vi "3D FIELD SWEEP with feedback, logging, both modes, starting step, and 1D sweep.vi"() -> ()   [LabVIEW 2018]
doc: "This example performs a serial port write and a serial port read. The parameters set for the serial port must match the parameters of the connected instrument or device. The VISA Configure Serial Port VI sets the configuration parameters. The front panel displays the controls used to configure the basic parameters, such as baud rate, data bits, and parity. The VI passes the VISA resource name to other VIs that perform operations on that VISA resource. The VISA Write function sends a command to the serial device and the VISA Read function returns data based on the command. The VISA Close function then closes the reference to the serial device. It is important to close the reference; otherwise, further communication through that port might not be possible."
uses:
  Program Files/National Instruments/LabVIEW 2018/examples/Instrument IO/Serial/support/Serial - Settings.ctl
  <vilib>/Instr/_visa.llb/VISA Configure Serial Port (Instr).vi
  <vilib>/Utility/file.llb/Write Delimited Spreadsheet (string).vi
panel:
  out "Magnetic field z [µT]":dbl
  out "Magnetic field y [µT]":dbl
  out "Magnetic field x [µT]":dbl
  out "Magnetic field strength [µT]":dbl
  in  "Direction field sweep":string(combo)
  in  "Minimum value B [µT]":dbl
  in  "Maximum value B [µT]":dbl
  in  "START":bool
  in  "Number of steps":dbl
  out "Current has stabilized":bool
  in  "Next iteration 2":bool
  in  "Starting step":dbl
  out "Current has stabilized":bool
  out "Current has stabilized":bool
  in  "Next iteration":bool
  in  "file path (use dialog)":path
  in  "Start":bool
  out "Start time 2":timestamp
  out "Angle \"phi\"":dbl
  out "Current iteration":i32
  in  "Number of steps":dbl
  in  "Angle theta [degrees]":dbl
  in  "Magnetic field strength [µT]":dbl
  in  "Octant":string(combo)
  in  "Sweep plane & fixed axis":string(combo)
  in  "OFF":bool
  in  "OK Button":bool
  in  "Magnetic field strength z [µT]":dbl
  in  "Magnetic field strength y [µT]":dbl
  in  "Magnetic field strength x [µT]":dbl
  in  "Static or field sweep?":string(combo)
  in  "Serial Settings":T1={"baud rate"=9600, "data bits"=8, "parity"=enum."None", "stop bits"=10, "flow control"=0} {"flow control" items=["None"=0, "XON/XOFF"=1, "RTS/CTS"=2, "DTR/DSR"=4]; "stop bits" items=["1.0"=10, "1.5"=15, "2.0"=20]; "data bits" min=5 max=8 step=1; "baud rate" items=["75"=75, "110"=110, "134"=134, "150"=150, "300"=300, "600"=600, "1200"=1200, "1800"=1800, "2400"=2400, "4800"=4800, "7200"=7200, "9600"=9600, "14400"=14400, "19200"=19200, "28800"=28800, "38400"=38400, "56000"=56000, "57600"=57600, "115200"=115200, "128000"=128000, "230400"=230400]}
  in  "VISA resource name":refnum<visa-resource-name>="COM1"
  # "Static field"
  # "1D magnitude sweep"
  # "Settings"
  # "3D field sweep"
  # "About the 3D field sweep"
  # "A onstant-magnitude, fixed-tilt, azimuthal sweep of a 3D vector is performed.\nThe mag,netic field vector is angled away from a fixed axis by a certain angle \"phi\". It then makes a circular motion around that fixed axis, eventually tracing out a full cone.\nYou choose a plane of variation ( x–y, x–z, or y–z) and hold one direction constant (e.g., z).  The sweep is performed clockwise, as seen from the origin."
  # "Must be a csv comma delimited excell file."
  # "How to connect the cables"
  # "Current state"
  # "Current state"
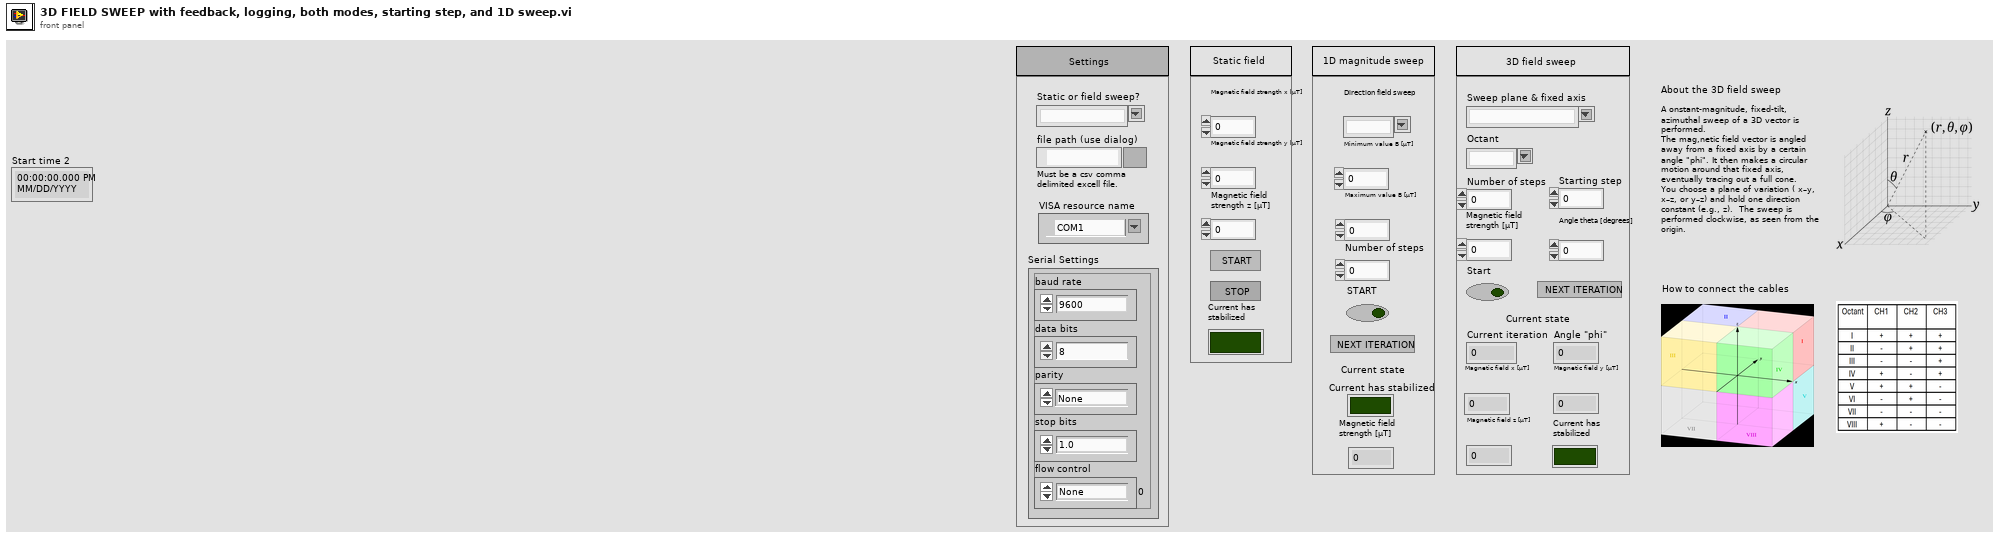
[diagram p1: front panel]
types:
  T1 = typedef "Serial - Settings.ctl" = cluster{"baud rate":u32, "data bits":u16, "parity":enum16{"None", "Odd", "Even", "Mark", "Space"}, "stop bits":u16, "flow control":u16}
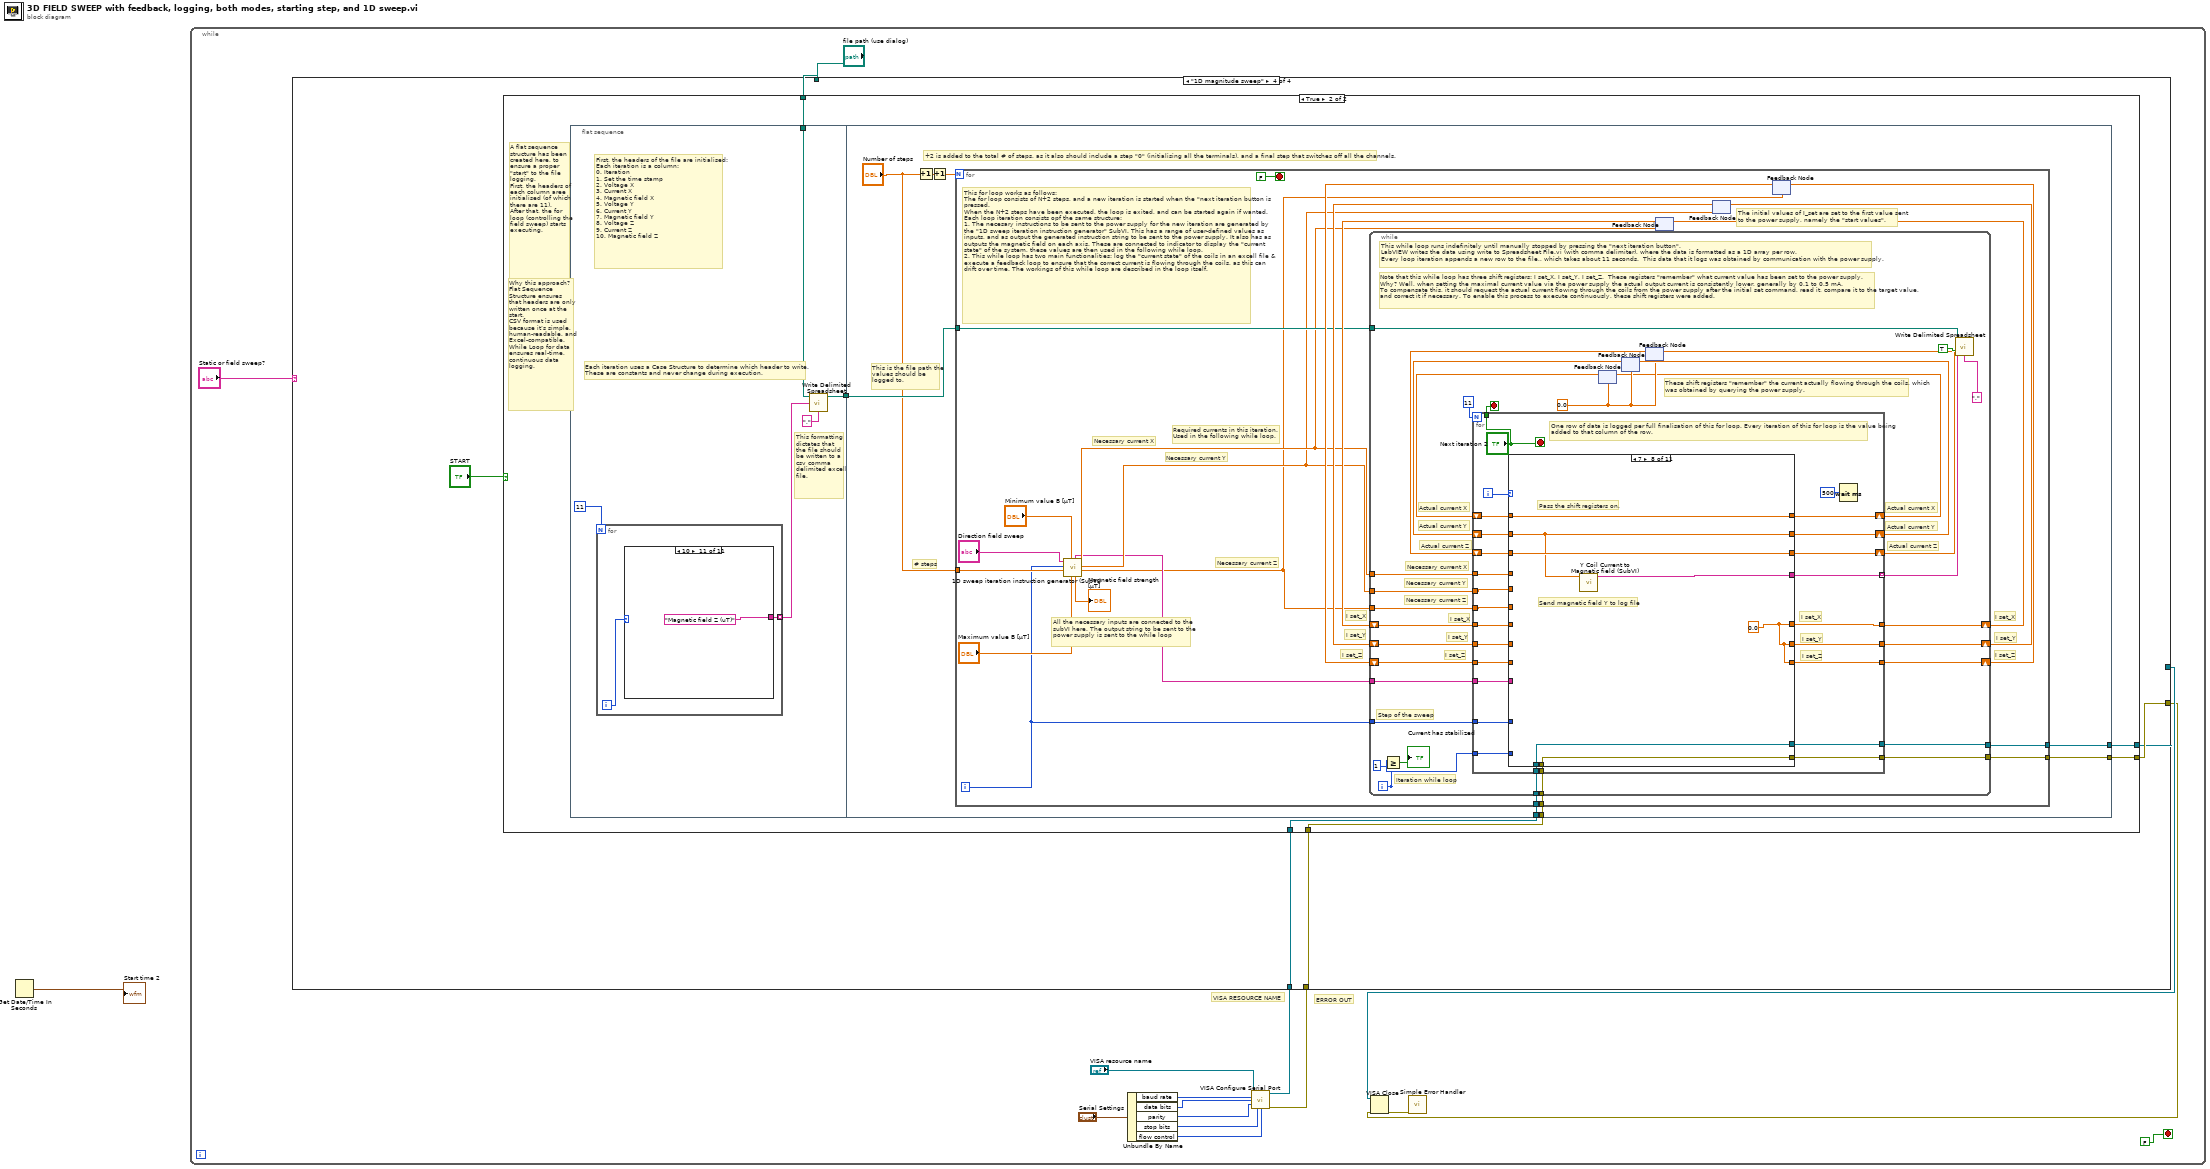
[diagram p0: block diagram]
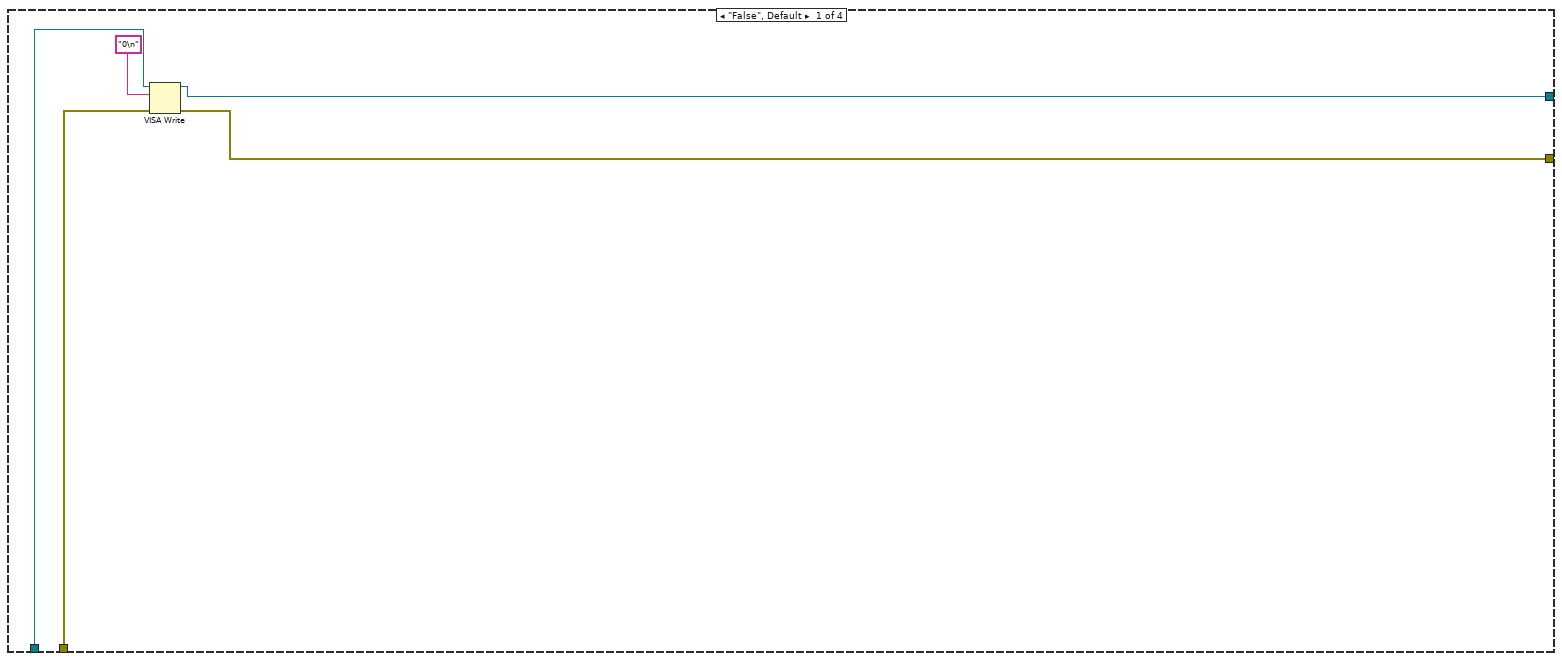
[diagram p2: hidden frame]
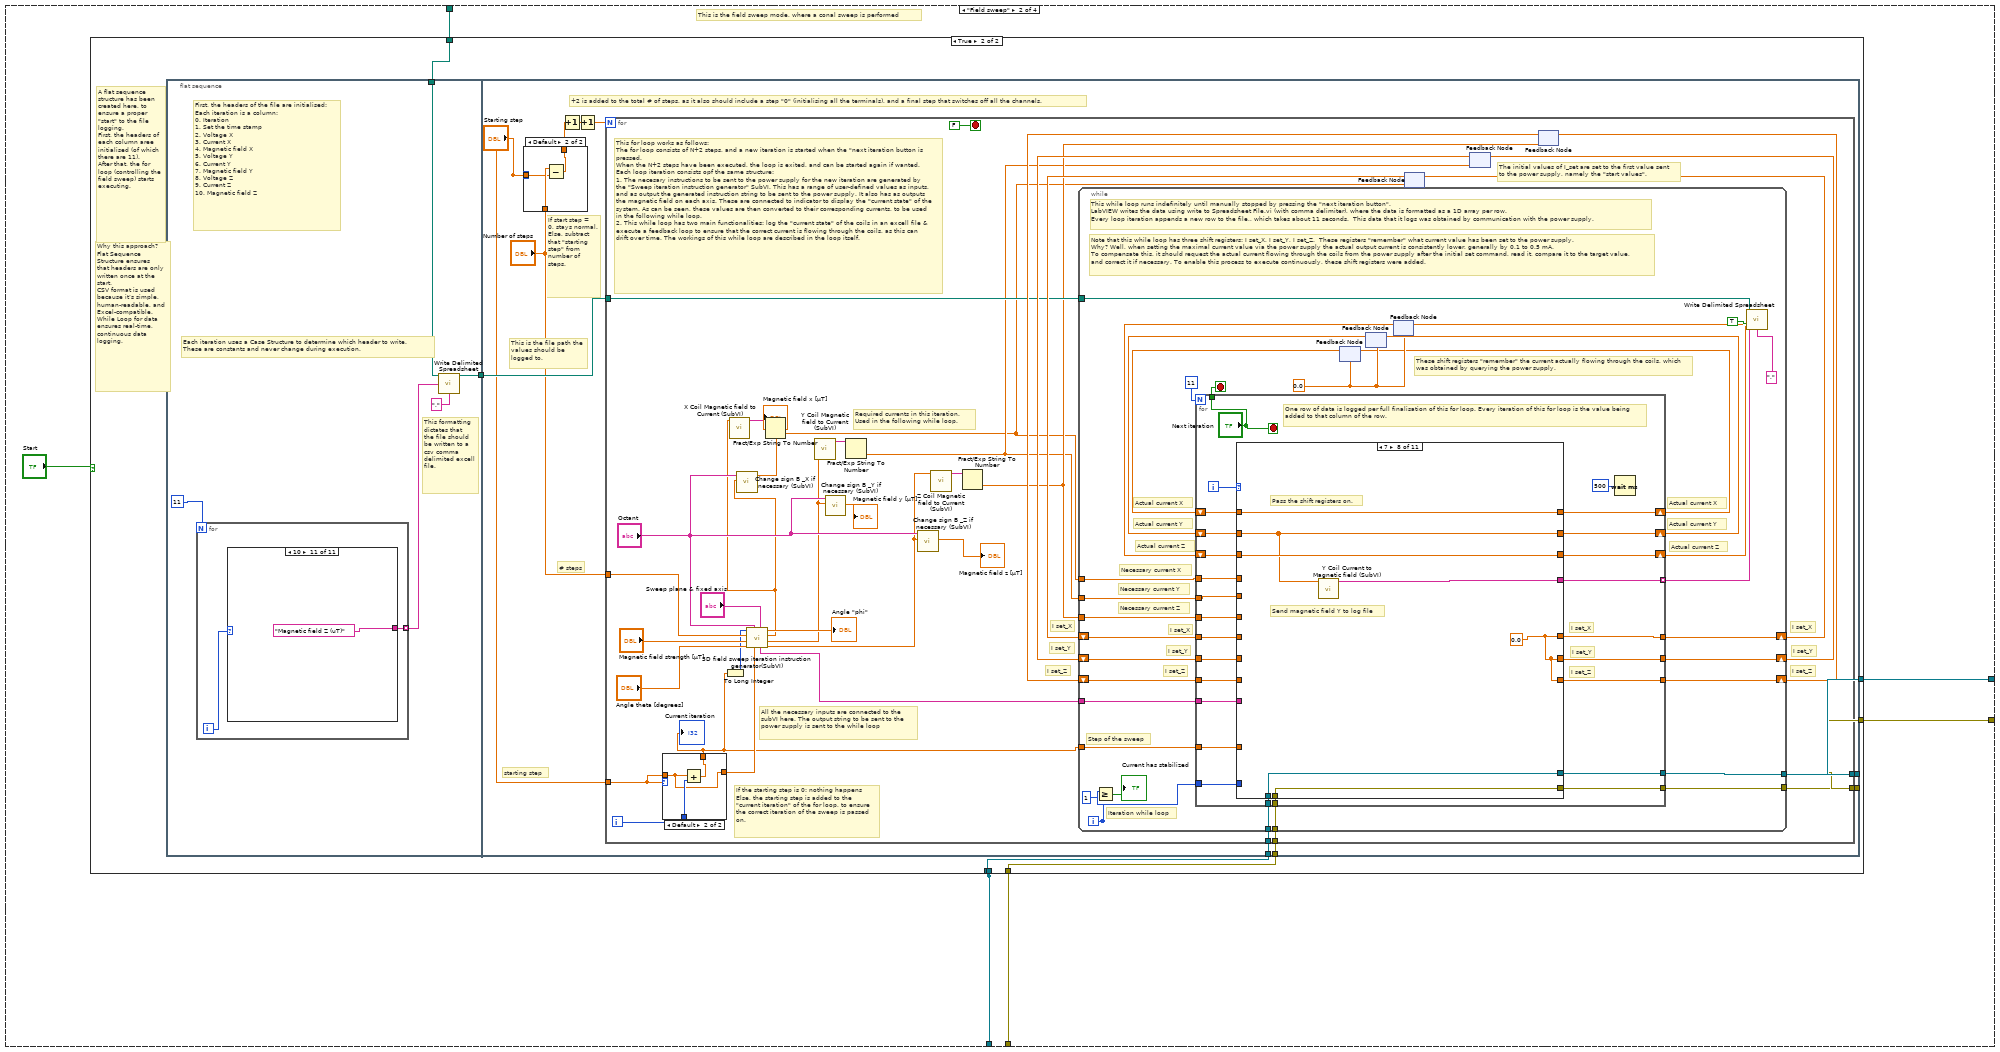
[diagram p3: hidden frame]
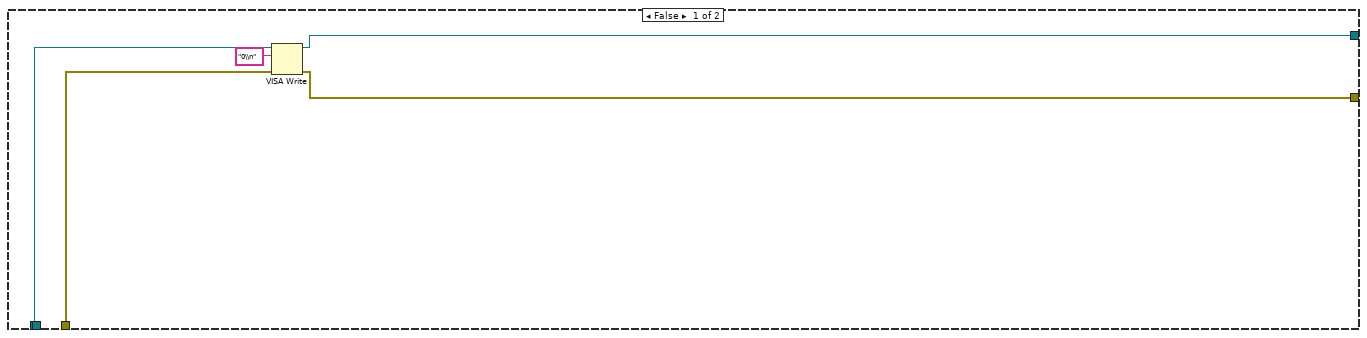
[diagram p4: hidden frame]
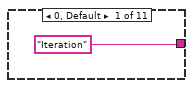
[diagram p5: hidden frame]
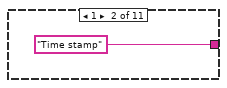
[diagram p6: hidden frame]
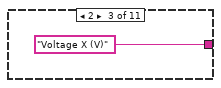
[diagram p7: hidden frame]
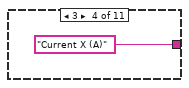
[diagram p8: hidden frame]
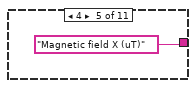
[diagram p9: hidden frame]
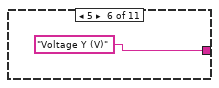
[diagram p10: hidden frame]
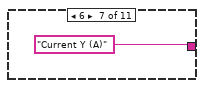
[diagram p11: hidden frame]
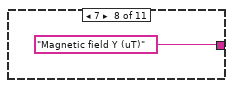
[diagram p12: hidden frame]
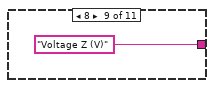
[diagram p13: hidden frame]
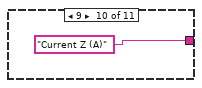
[diagram p14: hidden frame]
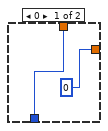
[diagram p16: hidden frame]
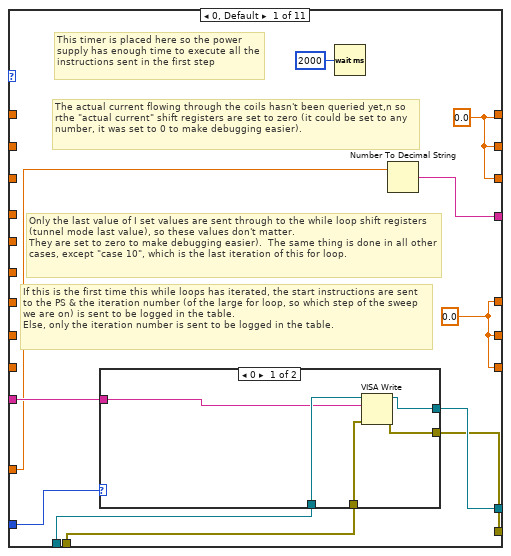
[diagram p17: hidden frame]
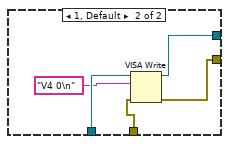
[diagram p18: hidden frame]
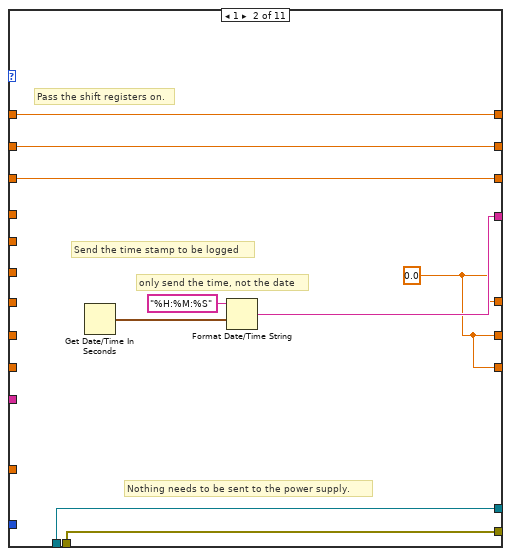
[diagram p19: hidden frame]
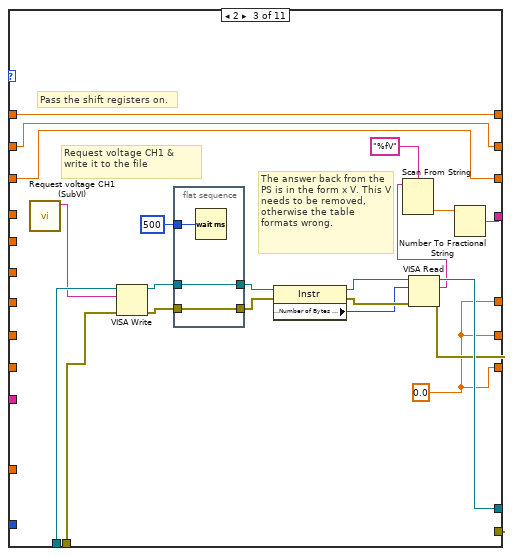
[diagram p20: hidden frame]
diagram:
  n1 = Get Date/Time In Seconds() -> (seconds since 1Jan1904=→"Start time 2":timestamp)
  n2 = while {
    stop <- FALSE stop-if-true
    # "VISA RESOURCE NAME"
    # "ERROR OUT"
    n3 = Unbundle By Name("Serial Settings") -> ("baud rate"=w13:u32, "data bits"=w2:u16, "parity"=w12:enum16{"None", "Odd", "Even", "Mark", "Space"}, "stop bits"=w11:u16, "flow control"=w10:u16)
    n4 = call-poly "VISA Configure Serial Port"("VISA resource name"="VISA resource name", "baud rate (9600)"=w13, "data bits (8)"=w2, "parity (0:none)"=w12, "stop bits (10: 1 bit)"=w11, "flow control (0:none)"=w10) -> ("VISA resource name out"=w3:refnum<visa-resource-name>, "error out"=w9:errorcluster)  [unwired: 3 in, 5 out]
    n5 = case shown="\"1D magnitude sweep\"" "Static or field sweep?" {
      tunnel: [w17 w26 w424 w793] -> w7
      tunnel: w3 -> [w19 w24 w421 w795]
      tunnel: w9 -> [w20 w25 w425 w794]
      tunnel: [w18 w27 w423 w792] -> w8
      tunnel: "file path (use dialog)" -> [_ w22 w420 w797]
      frame "False", Default {
        n6 = VISA Write(VISA resource name=w19, write buffer="0\n", error in (no error)=w20) -> (VISA resource name out=w18:refnum<visa-resource-name>, error out=w17:errorcluster)  [unwired: 1 out]
      }
      frame "Field sweep" {
        # "This is the field sweep mode, where a conal sweep is performed"
        n7 = case shown="True" "Start" {
          tunnel: [w32 w36] -> w27
          tunnel: [w31 w35] -> w26
          tunnel: w24 -> [w29 w38]
          tunnel: w25 -> [w30 w37]
          tunnel: w24 -> [_ _]
          tunnel: w22 -> [_ w33]
          frame False {
            n8 = VISA Write(VISA resource name=w29, write buffer="0\\n", error in (no error)=w30) -> (VISA resource name out=w32:refnum<visa-resource-name>, error out=w31:errorcluster)  [unwired: 1 out]
          }
          frame True {
            # "Why this approach?\nFlat Sequence Structure ensures that headers are only written once at the start.\nCSV format is used because it’s simple, human-readable, and Excel-compatible.\nWhile Loop for data ensures real-time, continuous data logging."
            # "A flat sequence structure has been created here, to ensure a proper \"start\" to the file logging. \nFirst, the headers of each column aree initialised (of which there are 11). \nAfter that, the for loop (controlling the field sweep) starts executing."
            n9 = flat-sequence {
              tunnel: w33 -> [w40]
              tunnel: [w39] -> w34
              tunnel: w38 -> [w64]
              tunnel: w37 -> [w63]
              tunnel: [w62] -> w36
              tunnel: [w61] -> w35
              tunnel: w34 -> [w60]
              frame #0 {
                # "Each iteration uses a Case Structure to determine which header to write.\nThese are constants and never change during execution."
                # "This formatting dictates that the file should be written to a csv comma delimited excell file."
                # "First, the headers of the file are initialised:\nEach iteration is a column:\n0. Iteration\n1. Set the time stamp\n2. Voltage X\n3. Current X\n4. Magnetic field X\n5. Voltage Y\n6. Current Y\n7. Magnetic field Y\n8. Voltage Z\n9. Current Z\n10. Magnetic field Z"
                n10 = for {
                  N: 11 -> [_]
                  tunnel: [w44] -> w42 mode=indexing
                  i -> [w45]
                  n11 = case shown="10" w45 {
                    tunnel: ["Iteration" "Time stamp" "Voltage X (V)" "Current X (A)" "Magnetic field X (uT)" "Voltage Y (V)" "Current Y (A)" "Magnetic field Y (uT)" "Voltage Z (V)" "Current Z (A)" "Magnetic field Z (uT)"] -> w44
                    frame 0, Default {
                    }
                    frame 1 {
                    }
                    frame 2 {
                    }
                    frame 3 {
                    }
                    frame 4 {
                    }
                    frame 5 {
                    }
                    frame 6 {
                    }
                    frame 7 {
                    }
                    frame 8 {
                    }
                    frame 9 {
                    }
                    frame 10 {
                    }
                  }
                }
                n12 = call-poly <vilib>:"Write Delimited Spreadsheet.vi"("file path (dialog if empty)"=w40, "1D data"=w42, "delimiter (\\t)"="," ("delimiter (\\t)")) -> ("new file path (Not A Path if cancelled)"=w39:path)  [unwired: 11 in, 1 out]
              }
              frame #1 {
                # "starting step"
                # "# steps"
                # "If start step = 0, stays normal.\nElse, subtract that \"starting step\" from number of steps."
                # "This is the file path the values should be logged to."
                # "+2 is added to the total # of steps, as it also should include a step \"0\" (initialising all the terminals), and a final step that switches off all the channels."
                n13 = case shown="Default" "Starting step" {
                  tunnel: "Number of steps" -> [w67 w70]
                  tunnel: [w67 w69] -> w58
                  tunnel: "Starting step" -> [_ w68]
                  frame 0 {
                  }
                  frame Default {
                    n14 = Subtract(x=w70, y=w68) -> (x-y=w69:dbl)
                  }
                }
                n15 = Increment(x=w58) -> (x+1=w66:dbl)
                n16 = Increment(x=w66) -> (x+1=w65:dbl)
                n17 = for {
                  N: w65 -> [_]
                  tunnel: "Number of steps" -> [w100]
                  tunnel: w64 -> [w91]
                  tunnel: w63 -> [w90]
                  tunnel: [w89] -> w62
                  tunnel: [w88] -> w61
                  tunnel: w60 -> [w87]
                  tunnel: "Starting step" -> [w79]
                  i -> [w80]
                  stop <- FALSE stop-if-true
                  # "If the starting step is 0: nothing happens\nElse, the starting step is added to the \"current iteration\" of the for loop, to ensure the correct iteration of the sweep is passed on."
                  # "The initial values of I_set are set to the first value sent to the power supply, namely the \"start values\"."
                  # "All the necessary inputs are connected to the subVI here. The output string to be sent to the power supply is sent to the while loop"
                  # "This for loop works as follows: \nThe for loop consists of N+2 steps, and a new iteration is started when the \"next iteration button is pressed.\nWhen the N+2 steps have been executed, the loop is exited, and can be started again if wanted.\nEach loop iteration consists opf the same structure:\n1. The necesary instructions to be sent to the power supply for the new iteration are generated by the \"Sweep iteration instruction generator\" SubVI. This has a range of user-defined values as inputs, and as output the generated instruction string to be sent to the power supply. It also has as outputs the magnetic field on each axis. These are connected to indicator to display the \"current state\" of the system. As can be seen, these values are then converted to their corresponding currents, to be used in the following while loop.\n2. This while loop has two main functionalities: log the \"current state\" of the coils in an excell file & execute a feedback loop to ensure that the correct current is flowing through the coils, as this can drift over time. The workings of this while loop are described in the loop itself."
                  # "I set_Z"
                  # "I set_Y"
                  # "I set_Y"
                  # "I set_Z"
                  # "I set_X"
                  # "I set_X"
                  # "Required currents in this iteration. \nUsed in the following while loop."
                  n18 = case shown="Default" w79 {
                    tunnel: w80 -> [w108 w111]
                    tunnel: [w108 w110] -> w73
                    tunnel: w79 -> [_ w109]
                    tunnel: [0 ("y") w109] -> w78
                    frame 0 {
                    }
                    frame Default {
                      n19 = Add(x=w109, y=w111) -> (x+y=w110:dbl)
                    }
                  }
                  "Current iteration" <- w73
                  n20 = To Long Integer(number=w73) -> (32bit integer=w72:i32)
                  n21 = call "3D field sweep iteration instruction generator(SubVI).vi"("Sweep plane & fixed axis"="Sweep plane & fixed axis", "Sweep starts later"=w78, "Octant"="Octant", "Angle theta [degrees]"="Angle theta [degrees]", "Magnetic field strength [µT]"="Magnetic field strength [µT]", "Number of steps"=w100, "Current iteration"=w72) -> ("Magnetic field z [µT]"=w74:dbl, "Magnetic field y [µT]"=w75:dbl, "Magnetic field x [µT]"=w76:dbl, "Azimuthal angle \"phi\""=→"Angle \"phi\"":dbl, "Output string instruction"=w92:string)
                  n22 = call "X Coil Magnetic field to Current (SubVI).vi"("Magnetic field [µT]"=w76) -> ("Current X"=w103:string)  [unwired: 10 in]
                  n23 = call "Change sign B _X if necessary (SubVI).vi"("Magnetic field x [µT] in"=w76, "Octant"="Octant") -> ("Magnetic field x [µT] out"=→"Magnetic field x [µT]":dbl)  [unwired: 9 in]
                  n24 = Fract/Exp String To Number(string=w103) -> (number=w81:dbl)  [unwired: 3 in, 1 out]
                  n25 = call "Y Coil Magnetic field to Current (SubVI).vi"("Magnetic field [µT]"=w75) -> ("Current Y"=w104:string)  [unwired: 10 in]
                  n26 = call "Change sign B _Y if necessary (SubVI).vi"("Magnetic field y [µT]  in"=w75, "Octant"="Octant") -> ("Magnetic field y [µT]  out"=→"Magnetic field y [µT]":dbl)  [unwired: 9 in]
                  n27 = Fract/Exp String To Number(string=w104) -> (number=w85:dbl)  [unwired: 3 in, 1 out]
                  n28 = call "Change sign B _Z if necessary (SubVI).vi"("Magnetic field z [µT] in"=w74, "Octant"="Octant") -> ("Magnetic field z [µT] out"=→"Magnetic field z [µT]":dbl)  [unwired: 9 in]
                  n29 = call "Z Coil Magnetic field to Current (SubVI).vi"("Magnetic field [µT]"=w74) -> ("Current Z"=w105:string)  [unwired: 10 in]
                  n30 = Fract/Exp String To Number(string=w105) -> (number=w86:dbl)  [unwired: 3 in, 1 out]
                  n31 = feedback #1(w81) -> (w98:dbl)
                  n32 = feedback #2(w85) -> (w95:dbl)
                  n33 = feedback #3(w86) -> (w93:dbl)
                  n34 = while {
                    tunnel: w87 -> [w139]
                    tunnel: w91 -> [w136]
                    tunnel: w90 -> [w135]
                    tunnel: [w134] -> w88
                    tunnel: [w133] -> w89
                    tunnel: w73 -> [w126]
                    shift-right: [w125] -> w97
                    shift-left: w98 -> [w124]
                    tunnel: w92 -> [w123]
                    shift-right: [w122] -> w96
                    shift-left: w95 -> [w120]
                    shift-right: [w121] -> w94
                    shift-left: w93 -> [w119]
                    tunnel: w81 -> [w118]
                    tunnel: w85 -> [w117]
                    tunnel: w86 -> [w116]
                    i -> [w115]
                    stop <- w112 stop-if-true
                    w128 = 0.0
                    # "These shift registers \"remember\" the current actually flowing through the coils, which was obtained by querying the power supply."
                    # "Note that this while loop has three shift registers: I set_X, I set_Y, I set_Z.  These registers \"remember\" what current value has been set to the power supply. \nWhy? Well, when setting the maximal current value via the power supply the actual output current is consistently lower, generally by 0.1 to 0.5 mA.\nTo compensate this, it should request the actual current flowing through the coils from the power supply after the initial set command, read it, compare it to the target value, and correct it if necessary. To enable this process to execute continuously, these shift registers were added."
                    # "This while loop runs indefinitely until manually stopped by pressing the \"next iteration button\". \nLabVIEW writes the data using write to Spreadsheet File.vi (with comma delimiter), where the data is formatted as a 1D array per row.\nEvery loop iteration appends a new row to the file,, which takes about 11 seconds.  This data that it logs was obtained by communication with the power supply."
                    # "Necessary current Z"
                    # "Necessary current Y"
                    # "Necessary current X"
                    # "I set_Z"
                    # "I set_Y"
                    # "Iteration while loop"
                    # "Step of the sweep"
                    # "I set_X"
                    # "Actual current Z"
                    # "Actual current Y"
                    # "Actual current X"
                    # "Actual current Z"
                    # "Actual current Y"
                    # "Actual current X"
                    n35 = Greater Or Equal?(x=w115, y=1) -> (x >= y?=→"Current has stabilized":bool)
                    n36 = feedback #4(w128) -> (w141:dbl)
                    n37 = feedback #5(w128) -> (w131:dbl)
                    n38 = feedback #6(w128) -> (w129:dbl)
                    n39 = for {
                      N: 11 -> [_]
                      tunnel: [w166] -> w140 mode=indexing
                      shift-right: [w161] -> w127
                      shift-left: w141 -> [w168]
                      tunnel: w136 -> [w165]
                      tunnel: w135 -> [w164]
                      tunnel: [w163] -> w134
                      tunnel: [w162] -> w133
                      shift-right: [w158] -> w132
                      shift-left: w131 -> [w160]
                      shift-right: [w157] -> w130
                      shift-left: w129 -> [w159]
                      tunnel: w115 -> [w156]
                      tunnel: w126 -> [w155]
                      tunnel: w124 -> [w154]
                      tunnel: [w153] -> w125
                      tunnel: w123 -> [w152]
                      tunnel: [w151] -> w122
                      tunnel: [w150] -> w121
                      tunnel: w120 -> [w149]
                      tunnel: w119 -> [w148]
                      tunnel: w118 -> [w147]
                      tunnel: w117 -> [w146]
                      tunnel: w116 -> [w145]
                      tunnel: ["Next iteration"] -> w112
                      i -> [w167]
                      stop <- "Next iteration" stop-if-true
                      # "One row of data is logged per full finalisation of this for loop. Every iteration of this for loop is the value being added to that column of the row."
                      # "I set_Y"
                      # "I set_Z"
                      # "I set_X"
                      n40 = case shown="7" w167 {
                        tunnel: [w173 w196 w200 w227 w249 w259 w278 w301 w313 w336 w373] -> w166
                        tunnel: w165 -> [w176 w195 w215 w236 w251 w261 w285 w305 w315 w340 w366]
                        tunnel: w164 -> [w177 w194 w214 w237 w250 w260 w286 w306 w314 w339 w365]
                        tunnel: [w179 w195 w213 w239 w251 w255 w283 w305 w312 w338 w368] -> w162
                        tunnel: [w178 w194 w212 w238 w250 w254 w282 w306 w311 w337 w367] -> w163
                        tunnel: [w175 w193 w219 w228 w252 w258 w280 w304 w310 w335 w372] -> w161
                        tunnel: w168 -> [_ w193 w219 _ w252 w258 w280 w304 w310 w335 w372]
                        tunnel: w160 -> [_ w192 w203 w225 w248 w257 _ w302 w309 w334 w364]
                        tunnel: w159 -> [_ w191 w202 w224 w247 w256 w279 w303 w308 _ w360]
                        tunnel: [w175 w192 w203 w225 w248 w257 w281 w302 w309 w334 w364] -> w158
                        tunnel: [w175 w191 w202 w224 w247 w256 w279 w303 w308 w333 w360] -> w157
                        tunnel: w156 -> [w174 _ _ _ _ _ _ _ _ _ w355]
                        tunnel: w155 -> [w170 _ _ _ _ _ _ _ _ _ _]
                        tunnel: [w171 w190 w199 w223 w246 w253 w277 w300 w307 w332 w369] -> w153
                        tunnel: w154 -> [_ _ _ _ _ _ _ _ _ _ w371]
                        tunnel: w152 -> [w172 _ _ _ _ _ _ _ _ _ _]
                        tunnel: [w171 w190 w199 w223 w246 w253 w277 w300 w307 w332 w361] -> w151
                        tunnel: [w171 w190 w199 w223 w246 w253 w277 w300 w307 w332 w357] -> w150
                        tunnel: w149 -> [_ _ _ _ _ _ _ _ _ _ w363]
                        tunnel: w148 -> [_ _ _ _ _ _ _ _ _ _ w358]
                        tunnel: w147 -> [_ _ _ _ _ _ _ _ _ _ w370]
                        tunnel: w146 -> [_ _ _ _ _ _ _ _ _ _ w362]
                        tunnel: w145 -> [_ _ _ _ _ _ _ _ _ _ w359]
                        frame 0, Default {
                          w171 = 0.0
                          w175 = 0.0
                          # "This timer is placed here so the power supply has enough time to execute all the instructions sent in the first step"
                          # "Only the last value of I set values are sent through to the while loop shift registers (tunnel mode last value), so these values don't matter. \nThey are set to zero to make debugging easier).  The same thing is done in all other cases, except \"case 10\", which is the last iteration of this for loop."
                          # "The actual current flowing through the coils hasn't been queried yet,n so rthe \"actual current\" shift registers are set to zero (it could be set to any number, it was set to 0 to make debugging easier)."
                          # "If this is the first time this while loops has iterated, the start instructions are sent to the PS & the iteration number (of the large for loop, so which step of the sweep we are on) is sent to be logged in the table.\nElse, only the iteration number is sent to be logged in the table."
                          n41 = case shown="0" w174 {
                            tunnel: [w184 w189] -> w179
                            tunnel: [w183 w188] -> w178
                            tunnel: w177 -> [w182 w187]
                            tunnel: w176 -> [w181 w186]
                            tunnel: w172 -> [w180 _]
                            frame 0 {
                              n42 = VISA Write(VISA resource name=w181, write buffer=w180, error in (no error)=w182) -> (VISA resource name out=w184:refnum<visa-resource-name>, error out=w183:errorcluster)  [unwired: 1 out]
                            }
                            frame 1, Default {
                              n43 = VISA Write(VISA resource name=w186, write buffer="V4 0\n", error in (no error)=w187) -> (VISA resource name out=w189:refnum<visa-resource-name>, error out=w188:errorcluster)  [unwired: 1 out]
                            }
                          }
                          n44 = Wait (ms)(milliseconds to wait=u32 2000) -> ()  [unwired: 1 out]
                          n45 = Number To Decimal String(number=w170) -> (decimal integer string=w173:string)  [unwired: 1 in]
                        }
                        frame 1 {
                          w190 = 0.0
                          # "Nothing needs to be sent to the power supply."
                          # "Pass the shift registers on."
                          # "only send the time, not the date"
                          # "Send the time stamp to be logged"
                          n46 = Get Date/Time In Seconds() -> (seconds since 1Jan1904=w198:timestamp)
                          n47 = Format Date/Time String(time format string (%c)="%H:%M:%S", seconds (now)=w198) -> (date/time string=w196:string)  [unwired: 1 in]
                        }
                        frame 2 {
                          w199 = 0.0
                          # "Pass the shift registers on."
                          # "The answer back from the PS is in the form x V. This V needs to be removed, otherwise the table formats wrong."
                          # "Request voltage CH1 & write it to the file"
                          n48 = call "Request voltage CH1 (SubVI).vi"() -> ("Request voltage CH1 / X"=w205:string)  [unwired: 11 in]
                          n49 = VISA Write(VISA resource name=w215, write buffer=w205, error in (no error)=w214) -> (VISA resource name out=w218:refnum<visa-resource-name>, error out=w217:errorcluster)  [unwired: 1 out]
                          n50 = flat-sequence {
                            tunnel: w217 -> [w220]
                            tunnel: w218 -> [w221]
                            tunnel: [w221] -> w211
                            tunnel: u32 500 ("delay before read (ms) static") -> [w222]
                            tunnel: [w220] -> w210
                            frame #0 {
                              n51 = Wait (ms)(milliseconds to wait=w222) -> ()  [unwired: 1 out]
                            }
                          }
                          n52 = property class="Instr"(reference=w211, error in=w210) -> (reference out=w209:refnum<visa-resource-name>, error out=w208:errorcluster, "Serial Settings:Number of Bytes at Serial Port"=w207:u32)
                          n53 = VISA Read(VISA resource name=w209, byte count=w207, error in (no error)=w208) -> (VISA resource name out=w213:refnum<visa-resource-name>, read buffer=w204:string, error out=w212:errorcluster)  [unwired: 1 out]
                          n54 = Scan From String(format string="%fV", input string=w204) -> (output 1=w201:dbl)  [unwired: 3 in, 3 out]
                          n55 = Number To Fractional String(number=w201) -> (F-format string=w200:string)  [unwired: 3 in]
                        }
                        frame 3 {
                          w223 = 0.0
                          # "Pass the shift registers on."
                          # "The answer back from the PS is in the form x A. This A needs to be removed, otherwise the table formats wrong."
                          # "Request current CH1; write it to the file; put it on the current X shift register"
                          n56 = call "Request current CH1(SubVI).vi"() -> ("Request current CH1 / X"=w229:string)  [unwired: 11 in]
                          n57 = VISA Write(VISA resource name=w236, write buffer=w229, error in (no error)=w237) -> (VISA resource name out=w242:refnum<visa-resource-name>, error out=w241:errorcluster)  [unwired: 1 out]
                          n58 = flat-sequence {
                            tunnel: w241 -> [w243]
                            tunnel: w242 -> [w244]
                            tunnel: [w244] -> w234
                            tunnel: u32 500 ("delay before read (ms) static") -> [w245]
                            tunnel: [w243] -> w233
                            frame #0 {
                              n59 = Wait (ms)(milliseconds to wait=w245) -> ()  [unwired: 1 out]
                            }
                          }
                          n60 = property class="Instr"(reference=w234, error in=w233) -> (reference out=w232:refnum<visa-resource-name>, error out=w230:errorcluster, "Serial Settings:Number of Bytes at Serial Port"=w231:u32)
                          n61 = VISA Read(VISA resource name=w232, byte count=w231, error in (no error)=w230) -> (VISA resource name out=w239:refnum<visa-resource-name>, read buffer=w235:string, error out=w238:errorcluster)  [unwired: 1 out]
                          n62 = Scan From String(format string="%fA", input string=w235) -> (output 1=w228:dbl)  [unwired: 3 in, 3 out]
                          n63 = Number To Fractional String(number=w228) -> (F-format string=w227:string)  [unwired: 3 in]
                        }
                        frame 4 {
                          w246 = 0.0
                          # "Pass the shift registers on."
                          # "Send magnetic field X to log file"
                          n64 = call "X Coil Current to Magnetic field (SubVI).vi"("Current X"=w252) -> ("Magnetic field X [µT]"=w249:string)  [unwired: 10 in]
                        }
                        frame 5 {
                          w253 = 0.0
                          # "Pass the shift registers on."
                          # "The answer back from the PS is in the form x V. This V needs to be removed, otherwise the table formats wrong."
                          # "Request voltage CH2 & write it to the file"
                          n65 = call "Request voltage CH2 (SubVI).vi"() -> ("Request voltage CH2 / Y"=w262:string)  [unwired: 11 in]
                          n66 = VISA Write(VISA resource name=w261, write buffer=w262, error in (no error)=w260) -> (VISA resource name out=w273:refnum<visa-resource-name>, error out=w272:errorcluster)  [unwired: 1 out]
                          n67 = flat-sequence {
                            tunnel: w272 -> [w274]
                            tunnel: w273 -> [w275]
                            tunnel: [w275] -> w270
                            tunnel: u32 500 ("delay before read (ms) static") -> [w276]
                            tunnel: [w274] -> w269
                            frame #0 {
                              n68 = Wait (ms)(milliseconds to wait=w276) -> ()  [unwired: 1 out]
                            }
                          }
                          n69 = property class="Instr"(reference=w270, error in=w269) -> (reference out=w268:refnum<visa-resource-name>, error out=w267:errorcluster, "Serial Settings:Number of Bytes at Serial Port"=w266:u32)
                          n70 = VISA Read(VISA resource name=w268, byte count=w266, error in (no error)=w267) -> (VISA resource name out=w255:refnum<visa-resource-name>, read buffer=w264:string, error out=w254:errorcluster)  [unwired: 1 out]
                          n71 = Scan From String(format string="%fV", input string=w264) -> (output 1=w263:dbl)  [unwired: 3 in, 3 out]
                          n72 = Number To Fractional String(number=w263) -> (F-format string=w259:string)  [unwired: 3 in]
                        }
                        frame 6 {
                          w277 = 0.0
                          # "Pass the shift registers on."
                          # "The answer back from the PS is in the form x A. This A needs to be removed, otherwise the table formats wrong."
                          # "Request current CH2; write it to the file; put it on the current Y shift register"
                          n73 = call "Request current CH2 (SubVI).vi"() -> ("Request current CH2 / Y"=w284:string)  [unwired: 11 in]
                          n74 = VISA Write(VISA resource name=w285, write buffer=w284, error in (no error)=w286) -> (VISA resource name out=w296:refnum<visa-resource-name>, error out=w295:errorcluster)  [unwired: 1 out]
                          n75 = flat-sequence {
                            tunnel: w295 -> [w297]
                            tunnel: w296 -> [w298]
                            tunnel: [w298] -> w292
                            tunnel: u32 500 ("delay before read (ms) static") -> [w299]
                            tunnel: [w297] -> w291
                            frame #0 {
                              n76 = Wait (ms)(milliseconds to wait=w299) -> ()  [unwired: 1 out]
                            }
                          }
                          n77 = property class="Instr"(reference=w292, error in=w291) -> (reference out=w290:refnum<visa-resource-name>, error out=w288:errorcluster, "Serial Settings:Number of Bytes at Serial Port"=w289:u32)
                          n78 = VISA Read(VISA resource name=w290, byte count=w289, error in (no error)=w288) -> (VISA resource name out=w283:refnum<visa-resource-name>, read buffer=w293:string, error out=w282:errorcluster)  [unwired: 1 out]
                          n79 = Scan From String(format string="%fA", input string=w293) -> (output 1=w281:dbl)  [unwired: 3 in, 3 out]
                          n80 = Number To Fractional String(number=w281) -> (F-format string=w278:string)  [unwired: 3 in]
                        }
                        frame 7 {
                          w300 = 0.0
                          # "Pass the shift registers on."
                          # "Send magnetic field Y to log file"
                          n81 = call "Y Coil Current to Magnetic field (SubVI).vi"("Current Y"=w302) -> ("Magnetic field Y [µT]"=w301:string)  [unwired: 10 in]
                        }
                        frame 8 {
                          w307 = 0.0
                          # "Pass the shift registers on."
                          # "The answer back from the PS is in the form x V. This V needs to be removed, otherwise the table formats wrong."
                          # "Request voltage CH3 & write it to the file"
                          n82 = call "Request voltage CH3 (SubVI).vi"() -> ("Request voltage CH3 / Z"=w316:string)  [unwired: 11 in]
                          n83 = VISA Write(VISA resource name=w315, write buffer=w316, error in (no error)=w314) -> (VISA resource name out=w327:refnum<visa-resource-name>, error out=w326:errorcluster)  [unwired: 1 out]
                          n84 = flat-sequence {
                            tunnel: w326 -> [w328]
                            tunnel: w327 -> [w329]
                            tunnel: [w329] -> w324
                            tunnel: u32 500 ("delay before read (ms) static") -> [w330]
                            tunnel: [w328] -> w323
                            frame #0 {
                              n85 = Wait (ms)(milliseconds to wait=w330) -> ()  [unwired: 1 out]
                            }
                          }
                          n86 = property class="Instr"(reference=w324, error in=w323) -> (reference out=w322:refnum<visa-resource-name>, error out=w321:errorcluster, "Serial Settings:Number of Bytes at Serial Port"=w320:u32)
                          n87 = VISA Read(VISA resource name=w322, byte count=w320, error in (no error)=w321) -> (VISA resource name out=w312:refnum<visa-resource-name>, read buffer=w318:string, error out=w311:errorcluster)  [unwired: 1 out]
                          n88 = Scan From String(format string="%fV", input string=w318) -> (output 1=w317:dbl)  [unwired: 3 in, 3 out]
                          n89 = Number To Fractional String(number=w317) -> (F-format string=w313:string)  [unwired: 3 in]
                        }
                        frame 9 {
                          w332 = 0.0
                          # "This timer was placed here because the entire for loop should take approximatly 10s and this timer ensures it. In the next for loop iteration the currents are corrected, but since that is not part of this log entry, it is done after this long wait statement."
                          # "Pass the shift registers on."
                          # "The answer back from the PS is in the form x A. This A needs to be removed, otherwise the table formats wrong."
                          # "Request current CH3; write it to the file; put it on the current Z shift register"
                          n90 = call "Request current CH3 (SubVI).vi"() -> ("Request current CH3 / Z"=w341:string)  [unwired: 11 in]
                          n91 = VISA Write(VISA resource name=w340, write buffer=w341, error in (no error)=w339) -> (VISA resource name out=w351:refnum<visa-resource-name>, error out=w350:errorcluster)  [unwired: 1 out]
                          n92 = flat-sequence {
                            tunnel: w350 -> [w352]
                            tunnel: w351 -> [w353]
                            tunnel: [w353] -> w347
                            tunnel: u32 500 ("delay before read (ms) static") -> [w354]
                            tunnel: [w352] -> w346
                            frame #0 {
                              n93 = Wait (ms)(milliseconds to wait=w354) -> ()  [unwired: 1 out]
                            }
                          }
                          n94 = property class="Instr"(reference=w347, error in=w346) -> (reference out=w345:refnum<visa-resource-name>, error out=w343:errorcluster, "Serial Settings:Number of Bytes at Serial Port"=w344:u32)
                          n95 = VISA Read(VISA resource name=w345, byte count=w344, error in (no error)=w343) -> (VISA resource name out=w338:refnum<visa-resource-name>, read buffer=w348:string, error out=w337:errorcluster)  [unwired: 1 out]
                          n96 = Scan From String(format string="%fA", input string=w348) -> (output 1=w333:dbl)  [unwired: 3 in, 3 out]
                          n97 = Wait (ms)(milliseconds to wait=u32 3000) -> ()  [unwired: 1 out]
                          n98 = Number To Fractional String(number=w333) -> (F-format string=w336:string)  [unwired: 3 in]
                        }
                        frame 10 {
                          # "This is set here to avoid overloading the loop & power supply."
                          # "Pass the shift registers on."
                          # "In the first iteration of this while loop, current correction is executed with the connections slightly different, because I set hasn't updated correctly yet, which would  lead to errosrs.\nI is checked if the current flowing through the coils is what it should be , and corrected if necessary."
                          # "Send magnetic field Z to log file"
                          n99 = case shown="Default" w355 {
                            tunnel: w372 -> [w378 w416]
                            tunnel: w371 -> [_ w415]
                            tunnel: w370 -> [w379 w414]
                            tunnel: [w386 w413] -> w369
                            tunnel: [w380 w411] -> w368
                            tunnel: [w381 w410] -> w367
                            tunnel: w366 -> [w383 w409]
                            tunnel: w365 -> [w382 w408]
                            tunnel: w364 -> [w376 w406]
                            tunnel: w363 -> [_ w405]
                            tunnel: w362 -> [w377 w404]
                            tunnel: [w385 w403] -> w361
                            tunnel: w360 -> [w374 w401]
                            tunnel: w359 -> [w375 w400]
                            tunnel: w358 -> [_ w399]
                            tunnel: [w384 w398] -> w357
                            frame 0 {
                              n100 = call "Corrected current calculator (SubVI).vi"("Necessary current"=w377, "I_set old"=w377, "Actual current"=w376) -> ("I_set new"=w385:dbl)  [unwired: 8 in]
                              n101 = call "Corrected current calculator (SubVI).vi"("Necessary current"=w379, "I_set old"=w379, "Actual current"=w378) -> ("I_set new"=w386:dbl)  [unwired: 8 in]
                              n102 = call "Corrected current calculator (SubVI).vi"("Necessary current"=w375, "I_set old"=w375, "Actual current"=w374) -> ("I_set new"=w384:dbl)  [unwired: 8 in]
                              n103 = Number To Fractional String(number=w386) -> (F-format string=w393:string)  [unwired: 3 in]
                              n104 = Number To Fractional String(number=w385) -> (F-format string=w391:string)  [unwired: 3 in]
                              n105 = Number To Fractional String(number=w384) -> (F-format string=w390:string)  [unwired: 3 in]
                              n106 = call "Set I2 (SubVI).vi"("Current Y"=w391) -> ("String"=w388:string)  [unwired: 10 in]
                              n107 = call "Set I1 (SubVI).vi"("Current X"=w393) -> ("String instruction"=w387:string)  [unwired: 10 in]
                              n108 = call "Set I3 (SubVI).vi"("Current Z"=w390) -> ("String"=w389:string)  [unwired: 10 in]
                              n109 = Concatenate Strings(w387, w388, w389) -> (w392:string)
                              n110 = VISA Write(VISA resource name=w383, write buffer=w392, error in (no error)=w382) -> (VISA resource name out=w380:refnum<visa-resource-name>, error out=w381:errorcluster)  [unwired: 1 out]
                            }
                            frame Default {
                              # "Correct currents: calculate the new necessary current value; send the new current value to the power supply; place this newt I set on the while loop shift register."
                              n111 = call "Corrected current calculator (SubVI).vi"("Necessary current"=w404, "I_set old"=w405, "Actual current"=w406) -> ("I_set new"=w403:dbl)  [unwired: 8 in]
                              n112 = call "Corrected current calculator (SubVI).vi"("Necessary current"=w414, "I_set old"=w415, "Actual current"=w416) -> ("I_set new"=w413:dbl)  [unwired: 8 in]
                              n113 = call "Corrected current calculator (SubVI).vi"("Necessary current"=w400, "I_set old"=w399, "Actual current"=w401) -> ("I_set new"=w398:dbl)  [unwired: 8 in]
                              n114 = Number To Fractional String(number=w413) -> (F-format string=w412:string)  [unwired: 3 in]
                              n115 = Number To Fractional String(number=w403) -> (F-format string=w402:string)  [unwired: 3 in]
                              n116 = Number To Fractional String(number=w398) -> (F-format string=w397:string)  [unwired: 3 in]
                              n117 = call "Set I2 (SubVI).vi"("Current Y"=w402) -> ("String"=w395:string)  [unwired: 10 in]
                              n118 = call "Set I1 (SubVI).vi"("Current X"=w412) -> ("String instruction"=w394:string)  [unwired: 10 in]
                              n119 = call "Set I3 (SubVI).vi"("Current Z"=w397) -> ("String"=w396:string)  [unwired: 10 in]
                              n120 = Concatenate Strings(w394, w395, w396) -> (w407:string)
                              n121 = VISA Write(VISA resource name=w409, write buffer=w407, error in (no error)=w408) -> (VISA resource name out=w411:refnum<visa-resource-name>, error out=w410:errorcluster)  [unwired: 1 out]
                            }
                          }
                          n122 = call "Z Coil Current to Magnetic field (SubVI).vi"("Current Z"=w360) -> ("Magnetic field Z [µT]"=w373:string)  [unwired: 10 in]
                          n123 = Wait (ms)(milliseconds to wait=u32 1000) -> ()  [unwired: 1 out]
                        }
                      }
                      n124 = Wait (ms)(milliseconds to wait=u32 500) -> ()  [unwired: 1 out]
                    }
                    n125 = feedback-in #4(w127) -> ()
                    n126 = feedback-in #5(w132) -> ()
                    n127 = feedback-in #6(w130) -> ()
                    n128 = call-poly <vilib>:"Write Delimited Spreadsheet.vi"("file path (dialog if empty)"=w139, "1D data"=w140, "append to file? (new file:F)"=TRUE, "delimiter (\\t)"="," ("delimiter (\\t)")) -> ()  [unwired: 10 in, 2 out]
                  }
                  n129 = feedback-in #1(w97) -> ()
                  n130 = feedback-in #2(w96) -> ()
                  n131 = feedback-in #3(w94) -> ()
                }
              }
            }
          }
        }
      }
      frame "Static field" {
        n132 = case shown="True" "OK Button" {
          tunnel: w425 -> [w430 w442]
          tunnel: w421 -> [w429 w441]
          tunnel: [w428 w444] -> w424
          tunnel: [w427 w443] -> w423
          tunnel: "Magnetic field strength x [µT]" -> [_ w445]
          tunnel: "Magnetic field strength y [µT]" -> [_ _]
          tunnel: w420 -> [_ w448]
          tunnel: "Magnetic field strength z [µT]" -> [_ w447]
          tunnel: "Magnetic field strength y [µT]" -> [_ w446]
          frame False {
            # "If the stop button is pressed -> turn the channels off"
            n133 = local read "OFF"() -> (w426:bool)
            n134 = case shown="False" w426 {
              tunnel: w430 -> [w433 w440]
              tunnel: w429 -> [w432 w439]
              tunnel: [w435 w438] -> w428
              tunnel: [w434 w437] -> w427
              frame False {
                n135 = VISA Write(VISA resource name=w432, write buffer="0\n", error in (no error)=w433) -> (VISA resource name out=w434:refnum<visa-resource-name>, error out=w435:errorcluster)  [unwired: 1 out]
              }
              frame True {
                n136 = call "Turn channels off (subVI).vi"() -> ("String"=w436:string)  [unwired: 11 in]
                n137 = VISA Write(VISA resource name=w439, write buffer=w436, error in (no error)=w440) -> (VISA resource name out=w437:refnum<visa-resource-name>, error out=w438:errorcluster)  [unwired: 1 out]
              }
            }
          }
          frame True {
            # "Why this approach?\nFlat Sequence Structure ensures that headers are only written once at the start.\nCSV format is used because it’s simple, human-readable, and Excel-compatible.\nWhile Loop for data ensures real-time, continuous data logging."
            # "A flat sequence structure has been created here, to ensure a proper \"start\" to the file logging. \nFirst, the headers of each column aree initialised (of which there are 11). \nAfter that, the for loop (controlling the field sweep) starts executing."
            # "IF this mode is turned on:\nThe logging file is initialised. Then, the initial instructions are sent to the power supply: \n1. Set the initial values for the current\n2. Set the voltage limits\n3. Turn all the channels on\nAfter the initial currents are set, the script request the actual current from the power supply, reads it, compares it to the target value, and corrects it if necessary. \nThe current system state (which includes the iteration step, timestamp, voltage, current, and magnetic field strength for each coil) must be logged continuously at approximately 10-second intervals. Both the logging and feedback control processes run continuously after the new current values are sent, untill the stop button is pressed"
            n138 = flat-sequence {
              tunnel: w448 -> [w451]
              tunnel: [w450] -> w449
              tunnel: w441 -> [w486]
              tunnel: [w469] -> _
              tunnel: [w485] -> w443
              tunnel: w449 -> [w484]
              tunnel: w447 -> [w477]
              tunnel: w446 -> [w476]
              tunnel: w445 -> [w475]
              tunnel: [w470] -> w444
              tunnel: w442 -> [w469]
              frame #0 {
                # "Each iteration uses a Case Structure to determine which header to write.\nThese are constants and never change during execution."
                # "This formatting dictates that the file should be written to a csv comma delimited excell file."
                # "First, the headers of the file are initialised:\nEach iteration is a column:\n0. Iteration\n1. Set the time stamp\n2. Voltage X\n3. Current X\n4. Magnetic field X\n5. Voltage Y\n6. Current Y\n7. Magnetic field Y\n8. Voltage Z\n9. Current Z\n10. Magnetic field Z"
                n139 = for {
                  N: 11 -> [_]
                  tunnel: [w455] -> w453 mode=indexing
                  i -> [w456]
                  n140 = case shown="10" w456 {
                    tunnel: ["Iteration" "Time stamp" "Voltage X (V)" "Current X (A)" "Magnetic field X (uT)" "Voltage Y (V)" "Current Y (A)" "Magnetic field Y (uT)" "Voltage Z (V)" "Current Z (A)" "Magnetic field Z (uT)"] -> w455
                    frame 0, Default {
                    }
                    frame 1 {
                    }
                    frame 2 {
                    }
                    frame 3 {
                    }
                    frame 4 {
                    }
                    frame 5 {
                    }
                    frame 6 {
                    }
                    frame 7 {
                    }
                    frame 8 {
                    }
                    frame 9 {
                    }
                    frame 10 {
                    }
                  }
                }
                n141 = call-poly <vilib>:"Write Delimited Spreadsheet.vi"("file path (dialog if empty)"=w451, "1D data"=w453, "delimiter (\\t)"="," ("delimiter (\\t)")) -> ("new file path (Not A Path if cancelled)"=w450:path)  [unwired: 11 in, 1 out]
              }
              frame #1 {
                # "Necessary current Z"
                # "Necessary current Y"
                # "Necessary current X"
                # "The initial values of I_set are set to the first value sent to the power supply, namely the \"start values\"."
                # "I set_Z"
                # "I set_Y"
                # "I set_Y"
                # "I set_Z"
                # "I set_X"
                # "I set_X"
                n142 = call "Static field instruction generator (SubVI).vi"("Magnetic field strength z [µT]"=w477, "Magnetic field strength y [µT]"=w476, "Magnetic field strength x [µT]"=w475) -> ("Necessary current Y"=w472:dbl, "Necessary current X"=w473:dbl, "Necessary current Z"=w471:dbl, "String"=w474:string)  [unwired: 5 in]
                n143 = feedback #7(w473) -> (w483:dbl)
                n144 = feedback #8(w472) -> (w480:dbl)
                n145 = feedback #9(w471) -> (w478:dbl)
                n146 = while {
                  tunnel: w484 -> [w514]
                  tunnel: w486 -> [w511]
                  tunnel: w469 -> [w510]
                  tunnel: [w509] -> w470
                  tunnel: [w508] -> w485
                  tunnel: 0 -> [w501]
                  shift-right: [w500] -> w482
                  shift-left: w483 -> [w499]
                  tunnel: w474 -> [w498]
                  shift-right: [w497] -> w481
                  shift-left: w480 -> [w495]
                  shift-right: [w496] -> w479
                  shift-left: w478 -> [w494]
                  tunnel: w473 -> [w493]
                  tunnel: w472 -> [w492]
                  tunnel: w471 -> [w491]
                  i -> [w490]
                  stop <- "OFF" stop-if-true
                  w503 = 0.0
                  # "These shift registers \"remember\" the current actually flowing through the coils, which was obtained by querying the power supply."
                  # "Note that this while loop has three shift registers: I set_X, I set_Y, I set_Z.  These registers \"remember\" what current value has been set to the power supply. \nWhy? Well, when setting the maximal current value via the power supply the actual output current is consistently lower, generally by 0.1 to 0.5 mA.\nTo compensate this, it should request the actual current flowing through the coils from the power supply after the initial set command, read it, compare it to the target value, and correct it if necessary. To enable this process to execute continuously, these shift registers were added."
                  # "This while loop runs indefinitely until manually stopped by pressing the \"next iteration button\". \nLabVIEW writes the data using write to Spreadsheet File.vi (with comma delimiter), where the data is formatted as a 1D array per row.\nEvery loop iteration appends a new row to the file,, which takes about 11 seconds.  This data that it logs was obtained by communication with the power supply."
                  # "Necessary current Z"
                  # "Necessary current Y"
                  # "Necessary current X"
                  # "I set_Z"
                  # "I set_Y"
                  # "Iteration while loop"
                  # "Step of the sweep"
                  # "I set_X"
                  # "Actual current Z"
                  # "Actual current Y"
                  # "Actual current X"
                  # "Actual current Z"
                  # "Actual current Y"
                  # "Actual current X"
                  n147 = Greater Or Equal?(x=w490, y=1) -> (x >= y?=→"Current has stabilized":bool)
                  n148 = feedback #10(w503) -> (w516:dbl)
                  n149 = feedback #11(w503) -> (w506:dbl)
                  n150 = feedback #12(w503) -> (w504:dbl)
                  n151 = for {
                    N: 11 -> [_]
                    tunnel: [w540] -> w515 mode=indexing
                    shift-right: [w535] -> w502
                    shift-left: w516 -> [w542]
                    tunnel: "OFF" -> [w543]
                    tunnel: w511 -> [w539]
                    tunnel: w510 -> [w538]
                    tunnel: [w537] -> w509
                    tunnel: [w536] -> w508
                    shift-right: [w532] -> w507
                    shift-left: w506 -> [w534]
                    shift-right: [w531] -> w505
                    shift-left: w504 -> [w533]
                    tunnel: w490 -> [w530]
                    tunnel: w501 -> [w529]
                    tunnel: w499 -> [w528]
                    tunnel: [w527] -> w500
                    tunnel: w498 -> [w526]
                    tunnel: [w525] -> w497
                    tunnel: [w524] -> w496
                    tunnel: w495 -> [w523]
                    tunnel: w494 -> [w522]
                    tunnel: w493 -> [w521]
                    tunnel: w492 -> [w520]
                    tunnel: w491 -> [w519]
                    i -> [w541]
                    stop <- w543 stop-if-true
                    # "One row of data is logged per full finalisation of this for loop. Every iteration of this for loop is the value being added to that column of the row."
                    # "I set_Y"
                    # "I set_Z"
                    # "I set_X"
                    n152 = case shown="10" w541 {
                      tunnel: [w548 w571 w575 w602 w624 w634 w653 w676 w688 w711 w748] -> w540
                      tunnel: w539 -> [w551 w570 w590 w611 w626 w636 w660 w680 w690 w715 w741]
                      tunnel: w538 -> [w552 w569 w589 w612 w625 w635 w661 w681 w689 w714 w740]
                      tunnel: [w554 w570 w588 w614 w626 w630 w658 w680 w687 w713 w743] -> w536
                      tunnel: [w553 w569 w587 w613 w625 w629 w657 w681 w686 w712 w742] -> w537
                      tunnel: [w550 w568 w594 w603 w627 w633 w655 w679 w685 w710 w747] -> w535
                      tunnel: w542 -> [_ w568 w594 _ w627 w633 w655 w679 w685 w710 w747]
                      tunnel: w534 -> [_ w567 w578 w600 w623 w632 _ w677 w684 w709 w739]
                      tunnel: w533 -> [_ w566 w577 w599 w622 w631 w654 w678 w683 _ w735]
                      tunnel: [w550 w567 w578 w600 w623 w632 w656 w677 w684 w709 w739] -> w532
                      tunnel: [w550 w566 w577 w599 w622 w631 w654 w678 w683 w708 w735] -> w531
                      tunnel: w530 -> [w549 _ _ _ _ _ _ _ _ _ w730]
                      tunnel: w529 -> [w545 _ _ _ _ _ _ _ _ _ _]
                      tunnel: [w546 w565 w574 w598 w621 w628 w652 w675 w682 w707 w744] -> w527
                      tunnel: w528 -> [_ _ _ _ _ _ _ _ _ _ w746]
                      tunnel: w526 -> [w547 _ _ _ _ _ _ _ _ _ _]
                      tunnel: [w546 w565 w574 w598 w621 w628 w652 w675 w682 w707 w736] -> w525
                      tunnel: [w546 w565 w574 w598 w621 w628 w652 w675 w682 w707 w732] -> w524
                      tunnel: w523 -> [_ _ _ _ _ _ _ _ _ _ w738]
                      tunnel: w522 -> [_ _ _ _ _ _ _ _ _ _ w733]
                      tunnel: w521 -> [_ _ _ _ _ _ _ _ _ _ w745]
                      tunnel: w520 -> [_ _ _ _ _ _ _ _ _ _ w737]
                      tunnel: w519 -> [_ _ _ _ _ _ _ _ _ _ w734]
                      frame 0, Default {
                        w546 = 0.0
                        w550 = 0.0
                        # "Only the last value of I set values are sent through to the while loop shift registers (tunnel mode last value), so these values don't matter. \nThey are set to zero to make debugging easier).  The same thing is done in all other cases, except \"case 10\", which is the last iteration of this for loop."
                        # "The actual current flowing through the coils hasn't been queried yet,n so rthe \"actual current\" shift registers are set to zero (it could be set to any number, it was set to 0 to make debugging easier)."
                        # "If this is the first time this while loops has iterated, the start instructions are sent to the PS & the iteration number (of the large for loop, so which step of the sweep we are on) is sent to be logged in the table.\nElse, only the iteration number is sent to be logged in the table."
                        n153 = case shown="0" w549 {
                          tunnel: [w559 w564] -> w554
                          tunnel: [w558 w563] -> w553
                          tunnel: w552 -> [w557 w562]
                          tunnel: w551 -> [w556 w561]
                          tunnel: w547 -> [w555 _]
                          frame 0 {
                            n154 = VISA Write(VISA resource name=w556, write buffer=w555, error in (no error)=w557) -> (VISA resource name out=w559:refnum<visa-resource-name>, error out=w558:errorcluster)  [unwired: 1 out]
                          }
                          frame 1, Default {
                            n155 = VISA Write(VISA resource name=w561, write buffer="V4 0\n", error in (no error)=w562) -> (VISA resource name out=w564:refnum<visa-resource-name>, error out=w563:errorcluster)  [unwired: 1 out]
                          }
                        }
                        n156 = Wait (ms)(milliseconds to wait=u32 2000) -> ()  [unwired: 1 out]
                        n157 = Number To Decimal String(number=w545) -> (decimal integer string=w548:string)  [unwired: 1 in]
                      }
                      frame 1 {
                        w565 = 0.0
                        # "Nothing needs to be sent to the power supply."
                        # "Pass the shift registers on."
                        # "only send the time, not the date"
                        # "Send the time stamp to be logged"
                        n158 = Get Date/Time In Seconds() -> (seconds since 1Jan1904=w573:timestamp)
                        n159 = Format Date/Time String(time format string (%c)="%H:%M:%S", seconds (now)=w573) -> (date/time string=w571:string)  [unwired: 1 in]
                      }
                      frame 2 {
                        w574 = 0.0
                        # "Pass the shift registers on."
                        # "The answer back from the PS is in the form x V. This V needs to be removed, otherwise the table formats wrong."
                        # "Request voltage CH1 & write it to the file"
                        n160 = call "Request voltage CH1 (SubVI).vi"() -> ("Request voltage CH1 / X"=w580:string)  [unwired: 11 in]
                        n161 = VISA Write(VISA resource name=w590, write buffer=w580, error in (no error)=w589) -> (VISA resource name out=w593:refnum<visa-resource-name>, error out=w592:errorcluster)  [unwired: 1 out]
                        n162 = flat-sequence {
                          tunnel: w592 -> [w595]
                          tunnel: w593 -> [w596]
                          tunnel: [w596] -> w586
                          tunnel: u32 500 ("delay before read (ms) static") -> [w597]
                          tunnel: [w595] -> w585
                          frame #0 {
                            n163 = Wait (ms)(milliseconds to wait=w597) -> ()  [unwired: 1 out]
                          }
                        }
                        n164 = property class="Instr"(reference=w586, error in=w585) -> (reference out=w584:refnum<visa-resource-name>, error out=w583:errorcluster, "Serial Settings:Number of Bytes at Serial Port"=w582:u32)
                        n165 = VISA Read(VISA resource name=w584, byte count=w582, error in (no error)=w583) -> (VISA resource name out=w588:refnum<visa-resource-name>, read buffer=w579:string, error out=w587:errorcluster)  [unwired: 1 out]
                        n166 = Scan From String(format string="%fV", input string=w579) -> (output 1=w576:dbl)  [unwired: 3 in, 3 out]
                        n167 = Number To Fractional String(number=w576) -> (F-format string=w575:string)  [unwired: 3 in]
                      }
                      frame 3 {
                        w598 = 0.0
                        # "Pass the shift registers on."
                        # "The answer back from the PS is in the form x A. This A needs to be removed, otherwise the table formats wrong."
                        # "Request current CH1; write it to the file; put it on the current X shift register"
                        n168 = call "Request current CH1(SubVI).vi"() -> ("Request current CH1 / X"=w604:string)  [unwired: 11 in]
                        n169 = VISA Write(VISA resource name=w611, write buffer=w604, error in (no error)=w612) -> (VISA resource name out=w617:refnum<visa-resource-name>, error out=w616:errorcluster)  [unwired: 1 out]
                        n170 = flat-sequence {
                          tunnel: w616 -> [w618]
                          tunnel: w617 -> [w619]
                          tunnel: [w619] -> w609
                          tunnel: u32 500 ("delay before read (ms) static") -> [w620]
                          tunnel: [w618] -> w608
                          frame #0 {
                            n171 = Wait (ms)(milliseconds to wait=w620) -> ()  [unwired: 1 out]
                          }
                        }
                        n172 = property class="Instr"(reference=w609, error in=w608) -> (reference out=w607:refnum<visa-resource-name>, error out=w605:errorcluster, "Serial Settings:Number of Bytes at Serial Port"=w606:u32)
                        n173 = VISA Read(VISA resource name=w607, byte count=w606, error in (no error)=w605) -> (VISA resource name out=w614:refnum<visa-resource-name>, read buffer=w610:string, error out=w613:errorcluster)  [unwired: 1 out]
                        n174 = Scan From String(format string="%fA", input string=w610) -> (output 1=w603:dbl)  [unwired: 3 in, 3 out]
                        n175 = Number To Fractional String(number=w603) -> (F-format string=w602:string)  [unwired: 3 in]
                      }
                      frame 4 {
                        w621 = 0.0
                        # "Pass the shift registers on."
                        # "Send magnetic field X to log file"
                        n176 = call "X Coil Current to Magnetic field (SubVI).vi"("Current X"=w627) -> ("Magnetic field X [µT]"=w624:string)  [unwired: 10 in]
                      }
                      frame 5 {
                        w628 = 0.0
                        # "Pass the shift registers on."
                        # "The answer back from the PS is in the form x V. This V needs to be removed, otherwise the table formats wrong."
                        # "Request voltage CH2 & write it to the file"
                        n177 = call "Request voltage CH2 (SubVI).vi"() -> ("Request voltage CH2 / Y"=w637:string)  [unwired: 11 in]
                        n178 = VISA Write(VISA resource name=w636, write buffer=w637, error in (no error)=w635) -> (VISA resource name out=w648:refnum<visa-resource-name>, error out=w647:errorcluster)  [unwired: 1 out]
                        n179 = flat-sequence {
                          tunnel: w647 -> [w649]
                          tunnel: w648 -> [w650]
                          tunnel: [w650] -> w645
                          tunnel: u32 500 ("delay before read (ms) static") -> [w651]
                          tunnel: [w649] -> w644
                          frame #0 {
                            n180 = Wait (ms)(milliseconds to wait=w651) -> ()  [unwired: 1 out]
                          }
                        }
                        n181 = property class="Instr"(reference=w645, error in=w644) -> (reference out=w643:refnum<visa-resource-name>, error out=w642:errorcluster, "Serial Settings:Number of Bytes at Serial Port"=w641:u32)
                        n182 = VISA Read(VISA resource name=w643, byte count=w641, error in (no error)=w642) -> (VISA resource name out=w630:refnum<visa-resource-name>, read buffer=w639:string, error out=w629:errorcluster)  [unwired: 1 out]
                        n183 = Scan From String(format string="%fV", input string=w639) -> (output 1=w638:dbl)  [unwired: 3 in, 3 out]
                        n184 = Number To Fractional String(number=w638) -> (F-format string=w634:string)  [unwired: 3 in]
                      }
                      frame 6 {
                        w652 = 0.0
                        # "Pass the shift registers on."
                        # "The answer back from the PS is in the form x A. This A needs to be removed, otherwise the table formats wrong."
                        # "Request current CH2; write it to the file; put it on the current Y shift register"
                        n185 = call "Request current CH2 (SubVI).vi"() -> ("Request current CH2 / Y"=w659:string)  [unwired: 11 in]
                        n186 = VISA Write(VISA resource name=w660, write buffer=w659, error in (no error)=w661) -> (VISA resource name out=w671:refnum<visa-resource-name>, error out=w670:errorcluster)  [unwired: 1 out]
                        n187 = flat-sequence {
                          tunnel: w670 -> [w672]
                          tunnel: w671 -> [w673]
                          tunnel: [w673] -> w667
                          tunnel: u32 500 ("delay before read (ms) static") -> [w674]
                          tunnel: [w672] -> w666
                          frame #0 {
                            n188 = Wait (ms)(milliseconds to wait=w674) -> ()  [unwired: 1 out]
                          }
                        }
                        n189 = property class="Instr"(reference=w667, error in=w666) -> (reference out=w665:refnum<visa-resource-name>, error out=w663:errorcluster, "Serial Settings:Number of Bytes at Serial Port"=w664:u32)
                        n190 = VISA Read(VISA resource name=w665, byte count=w664, error in (no error)=w663) -> (VISA resource name out=w658:refnum<visa-resource-name>, read buffer=w668:string, error out=w657:errorcluster)  [unwired: 1 out]
                        n191 = Scan From String(format string="%fA", input string=w668) -> (output 1=w656:dbl)  [unwired: 3 in, 3 out]
                        n192 = Number To Fractional String(number=w656) -> (F-format string=w653:string)  [unwired: 3 in]
                      }
                      frame 7 {
                        w675 = 0.0
                        # "Pass the shift registers on."
                        # "Send magnetic field Y to log file"
                        n193 = call "Y Coil Current to Magnetic field (SubVI).vi"("Current Y"=w677) -> ("Magnetic field Y [µT]"=w676:string)  [unwired: 10 in]
                      }
                      frame 8 {
                        w682 = 0.0
                        # "Pass the shift registers on."
                        # "The answer back from the PS is in the form x V. This V needs to be removed, otherwise the table formats wrong."
                        # "Request voltage CH3 & write it to the file"
                        n194 = call "Request voltage CH3 (SubVI).vi"() -> ("Request voltage CH3 / Z"=w691:string)  [unwired: 11 in]
                        n195 = VISA Write(VISA resource name=w690, write buffer=w691, error in (no error)=w689) -> (VISA resource name out=w702:refnum<visa-resource-name>, error out=w701:errorcluster)  [unwired: 1 out]
                        n196 = flat-sequence {
                          tunnel: w701 -> [w703]
                          tunnel: w702 -> [w704]
                          tunnel: [w704] -> w699
                          tunnel: u32 500 ("delay before read (ms) static") -> [w705]
                          tunnel: [w703] -> w698
                          frame #0 {
                            n197 = Wait (ms)(milliseconds to wait=w705) -> ()  [unwired: 1 out]
                          }
                        }
                        n198 = property class="Instr"(reference=w699, error in=w698) -> (reference out=w697:refnum<visa-resource-name>, error out=w696:errorcluster, "Serial Settings:Number of Bytes at Serial Port"=w695:u32)
                        n199 = VISA Read(VISA resource name=w697, byte count=w695, error in (no error)=w696) -> (VISA resource name out=w687:refnum<visa-resource-name>, read buffer=w693:string, error out=w686:errorcluster)  [unwired: 1 out]
                        n200 = Scan From String(format string="%fV", input string=w693) -> (output 1=w692:dbl)  [unwired: 3 in, 3 out]
                        n201 = Number To Fractional String(number=w692) -> (F-format string=w688:string)  [unwired: 3 in]
                      }
                      frame 9 {
                        w707 = 0.0
                        # "Pass the shift registers on."
                        # "The answer back from the PS is in the form x A. This A needs to be removed, otherwise the table formats wrong."
                        # "Request current CH3; write it to the file; put it on the current Z shift register"
                        n202 = call "Request current CH3 (SubVI).vi"() -> ("Request current CH3 / Z"=w716:string)  [unwired: 11 in]
                        n203 = VISA Write(VISA resource name=w715, write buffer=w716, error in (no error)=w714) -> (VISA resource name out=w726:refnum<visa-resource-name>, error out=w725:errorcluster)  [unwired: 1 out]
                        n204 = flat-sequence {
                          tunnel: w725 -> [w727]
                          tunnel: w726 -> [w728]
                          tunnel: [w728] -> w722
                          tunnel: u32 500 ("delay before read (ms) static") -> [w729]
                          tunnel: [w727] -> w721
                          frame #0 {
                            n205 = Wait (ms)(milliseconds to wait=w729) -> ()  [unwired: 1 out]
                          }
                        }
                        n206 = property class="Instr"(reference=w722, error in=w721) -> (reference out=w720:refnum<visa-resource-name>, error out=w718:errorcluster, "Serial Settings:Number of Bytes at Serial Port"=w719:u32)
                        n207 = Wait (ms)(milliseconds to wait=u32 3000) -> ()  [unwired: 1 out]
                        n208 = VISA Read(VISA resource name=w720, byte count=w719, error in (no error)=w718) -> (VISA resource name out=w713:refnum<visa-resource-name>, read buffer=w723:string, error out=w712:errorcluster)  [unwired: 1 out]
                        n209 = Scan From String(format string="%fA", input string=w723) -> (output 1=w708:dbl)  [unwired: 3 in, 3 out]
                        n210 = Number To Fractional String(number=w708) -> (F-format string=w711:string)  [unwired: 3 in]
                      }
                      frame 10 {
                        # "Pass the shift registers on."
                        # "In the first iteration of this while loop, current correction is executed with the connections slightly different, because I set hasn't updated correctly yet, which would  lead to errosrs.\nI is checked if the current flowing through the coils is what it should be , and corrected if necessary."
                        # "Send magnetic field Z to log file"
                        n211 = case shown="Default" w730 {
                          tunnel: w747 -> [w754 w791]
                          tunnel: w746 -> [_ w790]
                          tunnel: w745 -> [w753 w789]
                          tunnel: [w761 w788] -> w744
                          tunnel: [w758 w786] -> w743
                          tunnel: [w757 w785] -> w742
                          tunnel: w741 -> [w755 w784]
                          tunnel: w740 -> [w756 w783]
                          tunnel: w739 -> [w752 w781]
                          tunnel: w738 -> [_ w780]
                          tunnel: w737 -> [w751 w779]
                          tunnel: [w760 w778] -> w736
                          tunnel: w735 -> [w750 w776]
                          tunnel: w734 -> [w749 w775]
                          tunnel: w733 -> [_ w774]
                          tunnel: [w759 w773] -> w732
                          frame 0 {
                            n212 = call "Corrected current calculator (SubVI).vi"("Necessary current"=w751, "I_set old"=w751, "Actual current"=w752) -> ("I_set new"=w760:dbl)  [unwired: 8 in]
                            n213 = call "Corrected current calculator (SubVI).vi"("Necessary current"=w753, "I_set old"=w753, "Actual current"=w754) -> ("I_set new"=w761:dbl)  [unwired: 8 in]
                            n214 = call "Corrected current calculator (SubVI).vi"("Necessary current"=w749, "I_set old"=w749, "Actual current"=w750) -> ("I_set new"=w759:dbl)  [unwired: 8 in]
                            n215 = Number To Fractional String(number=w761) -> (F-format string=w768:string)  [unwired: 3 in]
                            n216 = Number To Fractional String(number=w760) -> (F-format string=w766:string)  [unwired: 3 in]
                            n217 = Number To Fractional String(number=w759) -> (F-format string=w765:string)  [unwired: 3 in]
                            n218 = call "Set I2 (SubVI).vi"("Current Y"=w766) -> ("String"=w763:string)  [unwired: 10 in]
                            n219 = call "Set I1 (SubVI).vi"("Current X"=w768) -> ("String instruction"=w762:string)  [unwired: 10 in]
                            n220 = call "Set I3 (SubVI).vi"("Current Z"=w765) -> ("String"=w764:string)  [unwired: 10 in]
                            n221 = Concatenate Strings(w762, w763, w764) -> (w767:string)
                            n222 = VISA Write(VISA resource name=w755, write buffer=w767, error in (no error)=w756) -> (VISA resource name out=w758:refnum<visa-resource-name>, error out=w757:errorcluster)  [unwired: 1 out]
                          }
                          frame Default {
                            # "Correct currents: calculate the new necessary current value; send the new current value to the power supply; place this newt I set on the while loop shift register."
                            n223 = call "Corrected current calculator (SubVI).vi"("Necessary current"=w779, "I_set old"=w780, "Actual current"=w781) -> ("I_set new"=w778:dbl)  [unwired: 8 in]
                            n224 = call "Corrected current calculator (SubVI).vi"("Necessary current"=w789, "I_set old"=w790, "Actual current"=w791) -> ("I_set new"=w788:dbl)  [unwired: 8 in]
                            n225 = call "Corrected current calculator (SubVI).vi"("Necessary current"=w775, "I_set old"=w774, "Actual current"=w776) -> ("I_set new"=w773:dbl)  [unwired: 8 in]
                            n226 = Number To Fractional String(number=w788) -> (F-format string=w787:string)  [unwired: 3 in]
                            n227 = Number To Fractional String(number=w778) -> (F-format string=w777:string)  [unwired: 3 in]
                            n228 = Number To Fractional String(number=w773) -> (F-format string=w772:string)  [unwired: 3 in]
                            n229 = call "Set I2 (SubVI).vi"("Current Y"=w777) -> ("String"=w770:string)  [unwired: 10 in]
                            n230 = call "Set I1 (SubVI).vi"("Current X"=w787) -> ("String instruction"=w769:string)  [unwired: 10 in]
                            n231 = call "Set I3 (SubVI).vi"("Current Z"=w772) -> ("String"=w771:string)  [unwired: 10 in]
                            n232 = Concatenate Strings(w769, w770, w771) -> (w782:string)
                            n233 = VISA Write(VISA resource name=w784, write buffer=w782, error in (no error)=w783) -> (VISA resource name out=w786:refnum<visa-resource-name>, error out=w785:errorcluster)  [unwired: 1 out]
                          }
                        }
                        n234 = call "Z Coil Current to Magnetic field (SubVI).vi"("Current Z"=w735) -> ("Magnetic field Z [µT]"=w748:string)  [unwired: 10 in]
                        n235 = Wait (ms)(milliseconds to wait=u32 1000) -> ()  [unwired: 1 out]
                      }
                    }
                    n236 = Wait (ms)(milliseconds to wait=u32 500) -> ()  [unwired: 1 out]
                  }
                  n237 = feedback-in #10(w502) -> ()
                  n238 = feedback-in #11(w507) -> ()
                  n239 = feedback-in #12(w505) -> ()
                  n240 = call-poly <vilib>:"Write Delimited Spreadsheet.vi"("file path (dialog if empty)"=w514, "1D data"=w515, "append to file? (new file:F)"=TRUE, "delimiter (\\t)"="," ("delimiter (\\t)")) -> ()  [unwired: 10 in, 2 out]
                }
                n241 = feedback-in #7(w482) -> ()
                n242 = feedback-in #8(w481) -> ()
                n243 = feedback-in #9(w479) -> ()
              }
            }
          }
        }
      }
      frame "1D magnitude sweep" {
        n244 = case shown="True" "START" {
          tunnel: [w802 w803] -> w792
          tunnel: [w801 w806] -> w793
          tunnel: w795 -> [w799 w808]
          tunnel: w794 -> [w800 w807]
          tunnel: w797 -> [_ w804]
          frame False {
            n245 = VISA Write(VISA resource name=w799, write buffer="0\\n", error in (no error)=w800) -> (VISA resource name out=w802:refnum<visa-resource-name>, error out=w801:errorcluster)  [unwired: 1 out]
          }
          frame True {
            # "Why this approach?\nFlat Sequence Structure ensures that headers are only written once at the start.\nCSV format is used because it’s simple, human-readable, and Excel-compatible.\nWhile Loop for data ensures real-time, continuous data logging."
            # "A flat sequence structure has been created here, to ensure a proper \"start\" to the file logging. \nFirst, the headers of each column aree initialised (of which there are 11). \nAfter that, the for loop (controlling the field sweep) starts executing."
            n246 = flat-sequence {
              tunnel: w804 -> [w810]
              tunnel: [w809] -> w805
              tunnel: w808 -> [w832]
              tunnel: w807 -> [w831]
              tunnel: [w830] -> w803
              tunnel: [w829] -> w806
              tunnel: w805 -> [w828]
              frame #0 {
                # "Each iteration uses a Case Structure to determine which header to write.\nThese are constants and never change during execution."
                # "This formatting dictates that the file should be written to a csv comma delimited excell file."
                # "First, the headers of the file are initialised:\nEach iteration is a column:\n0. Iteration\n1. Set the time stamp\n2. Voltage X\n3. Current X\n4. Magnetic field X\n5. Voltage Y\n6. Current Y\n7. Magnetic field Y\n8. Voltage Z\n9. Current Z\n10. Magnetic field Z"
                n247 = for {
                  N: 11 -> [_]
                  tunnel: [w814] -> w812 mode=indexing
                  i -> [w815]
                  n248 = case shown="10" w815 {
                    tunnel: ["Iteration" "Time stamp" "Voltage X (V)" "Current X (A)" "Magnetic field X (uT)" "Voltage Y (V)" "Current Y (A)" "Magnetic field Y (uT)" "Voltage Z (V)" "Current Z (A)" "Magnetic field Z (uT)"] -> w814
                    frame 0, Default {
                    }
                    frame 1 {
                    }
                    frame 2 {
                    }
                    frame 3 {
                    }
                    frame 4 {
                    }
                    frame 5 {
                    }
                    frame 6 {
                    }
                    frame 7 {
                    }
                    frame 8 {
                    }
                    frame 9 {
                    }
                    frame 10 {
                    }
                  }
                }
                n249 = call-poly <vilib>:"Write Delimited Spreadsheet.vi"("file path (dialog if empty)"=w810, "1D data"=w812, "delimiter (\\t)"="," ("delimiter (\\t)")) -> ("new file path (Not A Path if cancelled)"=w809:path)  [unwired: 11 in, 1 out]
              }
              frame #1 {
                # "# steps"
                # "This is the file path the values should be logged to."
                # "+2 is added to the total # of steps, as it also should include a step \"0\" (initialising all the terminals), and a final step that switches off all the channels."
                n250 = Increment(x="Number of steps") -> (x+1=w834:dbl)
                n251 = Increment(x=w834) -> (x+1=w833:dbl)
                n252 = for {
                  N: w833 -> [_]
                  tunnel: "Number of steps" -> [w843]
                  tunnel: w832 -> [w849]
                  tunnel: w831 -> [w848]
                  tunnel: [w847] -> w830
                  tunnel: [w846] -> w829
                  tunnel: w828 -> [w845]
                  i -> [w835]
                  stop <- FALSE stop-if-true
                  # "All the necessary inputs are connected to the subVI here. The output string to be sent to the power supply is sent to the while loop"
                  # "Necessary current X"
                  # "Necessary current Y"
                  # "Necessary current Z"
                  # "The initial values of I_set are set to the first value sent to the power supply, namely the \"start values\"."
                  # "This for loop works as follows: \nThe for loop consists of N+2 steps, and a new iteration is started when the \"next iteration button is pressed.\nWhen the N+2 steps have been executed, the loop is exited, and can be started again if wanted.\nEach loop iteration consists opf the same structure:\n1. The necesary instructions to be sent to the power supply for the new iteration are generated by the \"1D sweep iteration instruction generator\" SubVI. This has a range of user-defined values as inputs, and as output the generated instruction string to be sent to the power supply. It also has as outputs the magnetic field on each axis. These are connected to indicator to display the \"current state\" of the system, these values are then used in the following while loop.\n2. This while loop has two main functionalities: log the \"current state\" of the coils in an excell file & execute a feedback loop to ensure that the correct current is flowing through the coils, as this can drift over time. The workings of this while loop are described in the loop itself."
                  # "I set_Z"
                  # "I set_Y"
                  # "I set_Y"
                  # "I set_Z"
                  # "I set_X"
                  # "I set_X"
                  # "Required currents in this iteration. \nUsed in the following while loop."
                  n253 = call "1D sweep iteration instruction generator (SubVI).vi"("Maximum value B [µT]"="Maximum value B [µT]", "Minimum value B [µT]"="Minimum value B [µT]", "Number of steps"=w843, "Current iteration"=w835, "Direction field sweep"="Direction field sweep") -> ("Current z [µT]"=w836:dbl, "Current y [µT]"=w838:dbl, "Current x [µT]"=w839:dbl, "Magnetic field strength"=→"Magnetic field strength [µT]":dbl, "String"=w837:string)  [unwired: 2 in]
                  n254 = feedback #13(w839) -> (w855:dbl)
                  n255 = feedback #14(w838) -> (w852:dbl)
                  n256 = feedback #15(w836) -> (w850:dbl)
                  n257 = while {
                    tunnel: w845 -> [w884]
                    tunnel: w849 -> [w881]
                    tunnel: w848 -> [w880]
                    tunnel: [w879] -> w846
                    tunnel: [w878] -> w847
                    shift-right: [w871] -> w854
                    shift-left: w855 -> [w870]
                    tunnel: w837 -> [w869]
                    shift-right: [w868] -> w853
                    shift-left: w852 -> [w866]
                    shift-right: [w867] -> w851
                    shift-left: w850 -> [w865]
                    tunnel: w839 -> [w864]
                    tunnel: w838 -> [w863]
                    tunnel: w836 -> [w862]
                    tunnel: w835 -> [w858]
                    i -> [w861]
                    stop <- w857 stop-if-true
                    w873 = 0.0
                    # "These shift registers \"remember\" the current actually flowing through the coils, which was obtained by querying the power supply."
                    # "Note that this while loop has three shift registers: I set_X, I set_Y, I set_Z.  These registers \"remember\" what current value has been set to the power supply. \nWhy? Well, when setting the maximal current value via the power supply the actual output current is consistently lower, generally by 0.1 to 0.5 mA.\nTo compensate this, it should request the actual current flowing through the coils from the power supply after the initial set command, read it, compare it to the target value, and correct it if necessary. To enable this process to execute continuously, these shift registers were added."
                    # "This while loop runs indefinitely until manually stopped by pressing the \"next iteration button\". \nLabVIEW writes the data using write to Spreadsheet File.vi (with comma delimiter), where the data is formatted as a 1D array per row.\nEvery loop iteration appends a new row to the file,, which takes about 11 seconds.  This data that it logs was obtained by communication with the power supply."
                    # "Necessary current Z"
                    # "Necessary current Y"
                    # "Necessary current X"
                    # "I set_Z"
                    # "I set_Y"
                    # "Iteration while loop"
                    # "Step of the sweep"
                    # "I set_X"
                    # "Actual current Z"
                    # "Actual current Y"
                    # "Actual current X"
                    # "Actual current Z"
                    # "Actual current Y"
                    # "Actual current X"
                    n258 = Greater Or Equal?(x=w861, y=1) -> (x >= y?=→"Current has stabilized":bool)
                    n259 = feedback #16(w873) -> (w886:dbl)
                    n260 = feedback #17(w873) -> (w876:dbl)
                    n261 = feedback #18(w873) -> (w874:dbl)
                    n262 = for {
                      N: 11 -> [_]
                      tunnel: [w911] -> w885 mode=indexing
                      shift-right: [w906] -> w872
                      shift-left: w886 -> [w913]
                      tunnel: w881 -> [w910]
                      tunnel: w880 -> [w909]
                      tunnel: [w908] -> w879
                      tunnel: [w907] -> w878
                      shift-right: [w903] -> w877
                      shift-left: w876 -> [w905]
                      shift-right: [w902] -> w875
                      shift-left: w874 -> [w904]
                      tunnel: w861 -> [w901]
                      tunnel: w858 -> [w900]
                      tunnel: w870 -> [w899]
                      tunnel: [w898] -> w871
                      tunnel: w869 -> [w897]
                      tunnel: [w896] -> w868
                      tunnel: [w895] -> w867
                      tunnel: w866 -> [w894]
                      tunnel: w865 -> [w893]
                      tunnel: w864 -> [w892]
                      tunnel: w863 -> [w891]
                      tunnel: w862 -> [w890]
                      tunnel: ["Next iteration 2"] -> w857
                      i -> [w912]
                      stop <- "Next iteration 2" stop-if-true
                      # "One row of data is logged per full finalisation of this for loop. Every iteration of this for loop is the value being added to that column of the row."
                      # "I set_Y"
                      # "I set_Z"
                      # "I set_X"
                      n263 = case shown="7" w912 {
                        tunnel: [w918 w941 w945 w972 w994 w1004 w1023 w1046 w1058 w1081 w1118] -> w911
                        tunnel: w910 -> [w921 w940 w960 w981 w996 w1006 w1030 w1050 w1060 w1085 w1111]
                        tunnel: w909 -> [w922 w939 w959 w982 w995 w1005 w1031 w1051 w1059 w1084 w1110]
                        tunnel: [w924 w940 w958 w984 w996 w1000 w1028 w1050 w1057 w1083 w1113] -> w907
                        tunnel: [w923 w939 w957 w983 w995 w999 w1027 w1051 w1056 w1082 w1112] -> w908
                        tunnel: [w920 w938 w964 w973 w997 w1003 w1025 w1049 w1055 w1080 w1117] -> w906
                        tunnel: w913 -> [_ w938 w964 _ w997 w1003 w1025 w1049 w1055 w1080 w1117]
                        tunnel: w905 -> [_ w937 w948 w970 w993 w1002 _ w1047 w1054 w1079 w1109]
                        tunnel: w904 -> [_ w936 w947 w969 w992 w1001 w1024 w1048 w1053 _ w1105]
                        tunnel: [w920 w937 w948 w970 w993 w1002 w1026 w1047 w1054 w1079 w1109] -> w903
                        tunnel: [w920 w936 w947 w969 w992 w1001 w1024 w1048 w1053 w1078 w1105] -> w902
                        tunnel: w901 -> [w919 _ _ _ _ _ _ _ _ _ w1100]
                        tunnel: w900 -> [w915 _ _ _ _ _ _ _ _ _ _]
                        tunnel: [w916 w935 w944 w968 w991 w998 w1022 w1045 w1052 w1077 w1114] -> w898
                        tunnel: w899 -> [_ _ _ _ _ _ _ _ _ _ w1116]
                        tunnel: w897 -> [w917 _ _ _ _ _ _ _ _ _ _]
                        tunnel: [w916 w935 w944 w968 w991 w998 w1022 w1045 w1052 w1077 w1106] -> w896
                        tunnel: [w916 w935 w944 w968 w991 w998 w1022 w1045 w1052 w1077 w1102] -> w895
                        tunnel: w894 -> [_ _ _ _ _ _ _ _ _ _ w1108]
                        tunnel: w893 -> [_ _ _ _ _ _ _ _ _ _ w1103]
                        tunnel: w892 -> [_ _ _ _ _ _ _ _ _ _ w1115]
                        tunnel: w891 -> [_ _ _ _ _ _ _ _ _ _ w1107]
                        tunnel: w890 -> [_ _ _ _ _ _ _ _ _ _ w1104]
                        frame 0, Default {
                          w916 = 0.0
                          w920 = 0.0
                          # "This timer is placed here so the power supply has enough time to execute all the instructions sent in the first step"
                          # "Only the last value of I set values are sent through to the while loop shift registers (tunnel mode last value), so these values don't matter. \nThey are set to zero to make debugging easier).  The same thing is done in all other cases, except \"case 10\", which is the last iteration of this for loop."
                          # "The actual current flowing through the coils hasn't been queried yet,n so rthe \"actual current\" shift registers are set to zero (it could be set to any number, it was set to 0 to make debugging easier)."
                          # "If this is the first time this while loops has iterated, the start instructions are sent to the PS & the iteration number (of the large for loop, so which step of the sweep we are on) is sent to be logged in the table.\nElse, only the iteration number is sent to be logged in the table."
                          n264 = case shown="0" w919 {
                            tunnel: [w929 w934] -> w924
                            tunnel: [w928 w933] -> w923
                            tunnel: w922 -> [w927 w932]
                            tunnel: w921 -> [w926 w931]
                            tunnel: w917 -> [w925 _]
                            frame 0 {
                              n265 = VISA Write(VISA resource name=w926, write buffer=w925, error in (no error)=w927) -> (VISA resource name out=w929:refnum<visa-resource-name>, error out=w928:errorcluster)  [unwired: 1 out]
                            }
                            frame 1, Default {
                              n266 = VISA Write(VISA resource name=w931, write buffer="V4 0\n", error in (no error)=w932) -> (VISA resource name out=w934:refnum<visa-resource-name>, error out=w933:errorcluster)  [unwired: 1 out]
                            }
                          }
                          n267 = Wait (ms)(milliseconds to wait=u32 2000) -> ()  [unwired: 1 out]
                          n268 = Number To Decimal String(number=w915) -> (decimal integer string=w918:string)  [unwired: 1 in]
                        }
                        frame 1 {
                          w935 = 0.0
                          # "Nothing needs to be sent to the power supply."
                          # "Pass the shift registers on."
                          # "only send the time, not the date"
                          # "Send the time stamp to be logged"
                          n269 = Get Date/Time In Seconds() -> (seconds since 1Jan1904=w943:timestamp)
                          n270 = Format Date/Time String(time format string (%c)="%H:%M:%S", seconds (now)=w943) -> (date/time string=w941:string)  [unwired: 1 in]
                        }
                        frame 2 {
                          w944 = 0.0
                          # "Pass the shift registers on."
                          # "The answer back from the PS is in the form x V. This V needs to be removed, otherwise the table formats wrong."
                          # "Request voltage CH1 & write it to the file"
                          n271 = call "Request voltage CH1 (SubVI).vi"() -> ("Request voltage CH1 / X"=w950:string)  [unwired: 11 in]
                          n272 = VISA Write(VISA resource name=w960, write buffer=w950, error in (no error)=w959) -> (VISA resource name out=w963:refnum<visa-resource-name>, error out=w962:errorcluster)  [unwired: 1 out]
                          n273 = flat-sequence {
                            tunnel: w962 -> [w965]
                            tunnel: w963 -> [w966]
                            tunnel: [w966] -> w956
                            tunnel: u32 500 ("delay before read (ms) static") -> [w967]
                            tunnel: [w965] -> w955
                            frame #0 {
                              n274 = Wait (ms)(milliseconds to wait=w967) -> ()  [unwired: 1 out]
                            }
                          }
                          n275 = property class="Instr"(reference=w956, error in=w955) -> (reference out=w954:refnum<visa-resource-name>, error out=w953:errorcluster, "Serial Settings:Number of Bytes at Serial Port"=w952:u32)
                          n276 = VISA Read(VISA resource name=w954, byte count=w952, error in (no error)=w953) -> (VISA resource name out=w958:refnum<visa-resource-name>, read buffer=w949:string, error out=w957:errorcluster)  [unwired: 1 out]
                          n277 = Scan From String(format string="%fV", input string=w949) -> (output 1=w946:dbl)  [unwired: 3 in, 3 out]
                          n278 = Number To Fractional String(number=w946) -> (F-format string=w945:string)  [unwired: 3 in]
                        }
                        frame 3 {
                          w968 = 0.0
                          # "Pass the shift registers on."
                          # "The answer back from the PS is in the form x A. This A needs to be removed, otherwise the table formats wrong."
                          # "Request current CH1; write it to the file; put it on the current X shift register"
                          n279 = call "Request current CH1(SubVI).vi"() -> ("Request current CH1 / X"=w974:string)  [unwired: 11 in]
                          n280 = VISA Write(VISA resource name=w981, write buffer=w974, error in (no error)=w982) -> (VISA resource name out=w987:refnum<visa-resource-name>, error out=w986:errorcluster)  [unwired: 1 out]
                          n281 = flat-sequence {
                            tunnel: w986 -> [w988]
                            tunnel: w987 -> [w989]
                            tunnel: [w989] -> w979
                            tunnel: u32 500 ("delay before read (ms) static") -> [w990]
                            tunnel: [w988] -> w978
                            frame #0 {
                              n282 = Wait (ms)(milliseconds to wait=w990) -> ()  [unwired: 1 out]
                            }
                          }
                          n283 = property class="Instr"(reference=w979, error in=w978) -> (reference out=w977:refnum<visa-resource-name>, error out=w975:errorcluster, "Serial Settings:Number of Bytes at Serial Port"=w976:u32)
                          n284 = VISA Read(VISA resource name=w977, byte count=w976, error in (no error)=w975) -> (VISA resource name out=w984:refnum<visa-resource-name>, read buffer=w980:string, error out=w983:errorcluster)  [unwired: 1 out]
                          n285 = Scan From String(format string="%fA", input string=w980) -> (output 1=w973:dbl)  [unwired: 3 in, 3 out]
                          n286 = Number To Fractional String(number=w973) -> (F-format string=w972:string)  [unwired: 3 in]
                        }
                        frame 4 {
                          w991 = 0.0
                          # "Pass the shift registers on."
                          # "Send magnetic field X to log file"
                          n287 = call "X Coil Current to Magnetic field (SubVI).vi"("Current X"=w997) -> ("Magnetic field X [µT]"=w994:string)  [unwired: 10 in]
                        }
                        frame 5 {
                          w998 = 0.0
                          # "Pass the shift registers on."
                          # "The answer back from the PS is in the form x V. This V needs to be removed, otherwise the table formats wrong."
                          # "Request voltage CH2 & write it to the file"
                          n288 = call "Request voltage CH2 (SubVI).vi"() -> ("Request voltage CH2 / Y"=w1007:string)  [unwired: 11 in]
                          n289 = VISA Write(VISA resource name=w1006, write buffer=w1007, error in (no error)=w1005) -> (VISA resource name out=w1018:refnum<visa-resource-name>, error out=w1017:errorcluster)  [unwired: 1 out]
                          n290 = flat-sequence {
                            tunnel: w1017 -> [w1019]
                            tunnel: w1018 -> [w1020]
                            tunnel: [w1020] -> w1015
                            tunnel: u32 500 ("delay before read (ms) static") -> [w1021]
                            tunnel: [w1019] -> w1014
                            frame #0 {
                              n291 = Wait (ms)(milliseconds to wait=w1021) -> ()  [unwired: 1 out]
                            }
                          }
                          n292 = property class="Instr"(reference=w1015, error in=w1014) -> (reference out=w1013:refnum<visa-resource-name>, error out=w1012:errorcluster, "Serial Settings:Number of Bytes at Serial Port"=w1011:u32)
                          n293 = VISA Read(VISA resource name=w1013, byte count=w1011, error in (no error)=w1012) -> (VISA resource name out=w1000:refnum<visa-resource-name>, read buffer=w1009:string, error out=w999:errorcluster)  [unwired: 1 out]
                          n294 = Scan From String(format string="%fV", input string=w1009) -> (output 1=w1008:dbl)  [unwired: 3 in, 3 out]
                          n295 = Number To Fractional String(number=w1008) -> (F-format string=w1004:string)  [unwired: 3 in]
                        }
                        frame 6 {
                          w1022 = 0.0
                          # "Pass the shift registers on."
                          # "The answer back from the PS is in the form x A. This A needs to be removed, otherwise the table formats wrong."
                          # "Request current CH2; write it to the file; put it on the current Y shift register"
                          n296 = call "Request current CH2 (SubVI).vi"() -> ("Request current CH2 / Y"=w1029:string)  [unwired: 11 in]
                          n297 = VISA Write(VISA resource name=w1030, write buffer=w1029, error in (no error)=w1031) -> (VISA resource name out=w1041:refnum<visa-resource-name>, error out=w1040:errorcluster)  [unwired: 1 out]
                          n298 = flat-sequence {
                            tunnel: w1040 -> [w1042]
                            tunnel: w1041 -> [w1043]
                            tunnel: [w1043] -> w1037
                            tunnel: u32 500 ("delay before read (ms) static") -> [w1044]
                            tunnel: [w1042] -> w1036
                            frame #0 {
                              n299 = Wait (ms)(milliseconds to wait=w1044) -> ()  [unwired: 1 out]
                            }
                          }
                          n300 = property class="Instr"(reference=w1037, error in=w1036) -> (reference out=w1035:refnum<visa-resource-name>, error out=w1033:errorcluster, "Serial Settings:Number of Bytes at Serial Port"=w1034:u32)
                          n301 = VISA Read(VISA resource name=w1035, byte count=w1034, error in (no error)=w1033) -> (VISA resource name out=w1028:refnum<visa-resource-name>, read buffer=w1038:string, error out=w1027:errorcluster)  [unwired: 1 out]
                          n302 = Scan From String(format string="%fA", input string=w1038) -> (output 1=w1026:dbl)  [unwired: 3 in, 3 out]
                          n303 = Number To Fractional String(number=w1026) -> (F-format string=w1023:string)  [unwired: 3 in]
                        }
                        frame 7 {
                          w1045 = 0.0
                          # "Pass the shift registers on."
                          # "Send magnetic field Y to log file"
                          n304 = call "Y Coil Current to Magnetic field (SubVI).vi"("Current Y"=w1047) -> ("Magnetic field Y [µT]"=w1046:string)  [unwired: 10 in]
                        }
                        frame 8 {
                          w1052 = 0.0
                          # "Pass the shift registers on."
                          # "The answer back from the PS is in the form x V. This V needs to be removed, otherwise the table formats wrong."
                          # "Request voltage CH3 & write it to the file"
                          n305 = call "Request voltage CH3 (SubVI).vi"() -> ("Request voltage CH3 / Z"=w1061:string)  [unwired: 11 in]
                          n306 = VISA Write(VISA resource name=w1060, write buffer=w1061, error in (no error)=w1059) -> (VISA resource name out=w1072:refnum<visa-resource-name>, error out=w1071:errorcluster)  [unwired: 1 out]
                          n307 = flat-sequence {
                            tunnel: w1071 -> [w1073]
                            tunnel: w1072 -> [w1074]
                            tunnel: [w1074] -> w1069
                            tunnel: u32 500 ("delay before read (ms) static") -> [w1075]
                            tunnel: [w1073] -> w1068
                            frame #0 {
                              n308 = Wait (ms)(milliseconds to wait=w1075) -> ()  [unwired: 1 out]
                            }
                          }
                          n309 = property class="Instr"(reference=w1069, error in=w1068) -> (reference out=w1067:refnum<visa-resource-name>, error out=w1066:errorcluster, "Serial Settings:Number of Bytes at Serial Port"=w1065:u32)
                          n310 = VISA Read(VISA resource name=w1067, byte count=w1065, error in (no error)=w1066) -> (VISA resource name out=w1057:refnum<visa-resource-name>, read buffer=w1063:string, error out=w1056:errorcluster)  [unwired: 1 out]
                          n311 = Scan From String(format string="%fV", input string=w1063) -> (output 1=w1062:dbl)  [unwired: 3 in, 3 out]
                          n312 = Number To Fractional String(number=w1062) -> (F-format string=w1058:string)  [unwired: 3 in]
                        }
                        frame 9 {
                          w1077 = 0.0
                          # "This timer was placed here because the entire for loop should take approximatly 10s and this timer ensures it. In the next for loop iteration the currents are corrected, but since that is not part of this log entry, it is done after this long wait statement."
                          # "Pass the shift registers on."
                          # "The answer back from the PS is in the form x A. This A needs to be removed, otherwise the table formats wrong."
                          # "Request current CH3; write it to the file; put it on the current Z shift register"
                          n313 = call "Request current CH3 (SubVI).vi"() -> ("Request current CH3 / Z"=w1086:string)  [unwired: 11 in]
                          n314 = VISA Write(VISA resource name=w1085, write buffer=w1086, error in (no error)=w1084) -> (VISA resource name out=w1096:refnum<visa-resource-name>, error out=w1095:errorcluster)  [unwired: 1 out]
                          n315 = flat-sequence {
                            tunnel: w1095 -> [w1097]
                            tunnel: w1096 -> [w1098]
                            tunnel: [w1098] -> w1092
                            tunnel: u32 500 ("delay before read (ms) static") -> [w1099]
                            tunnel: [w1097] -> w1091
                            frame #0 {
                              n316 = Wait (ms)(milliseconds to wait=w1099) -> ()  [unwired: 1 out]
                            }
                          }
                          n317 = property class="Instr"(reference=w1092, error in=w1091) -> (reference out=w1090:refnum<visa-resource-name>, error out=w1088:errorcluster, "Serial Settings:Number of Bytes at Serial Port"=w1089:u32)
                          n318 = VISA Read(VISA resource name=w1090, byte count=w1089, error in (no error)=w1088) -> (VISA resource name out=w1083:refnum<visa-resource-name>, read buffer=w1093:string, error out=w1082:errorcluster)  [unwired: 1 out]
                          n319 = Scan From String(format string="%fA", input string=w1093) -> (output 1=w1078:dbl)  [unwired: 3 in, 3 out]
                          n320 = Wait (ms)(milliseconds to wait=u32 3000) -> ()  [unwired: 1 out]
                          n321 = Number To Fractional String(number=w1078) -> (F-format string=w1081:string)  [unwired: 3 in]
                        }
                        frame 10 {
                          # "This is set here to avoid overloading the loop & power supply."
                          # "Pass the shift registers on."
                          # "In the first iteration of this while loop, current correction is executed with the connections slightly different, because I set hasn't updated correctly yet, which would  lead to errosrs.\nI is checked if the current flowing through the coils is what it should be , and corrected if necessary."
                          # "Send magnetic field Z to log file"
                          n322 = case shown="Default" w1100 {
                            tunnel: w1117 -> [w1123 w1161]
                            tunnel: w1116 -> [_ w1160]
                            tunnel: w1115 -> [w1124 w1159]
                            tunnel: [w1131 w1158] -> w1114
                            tunnel: [w1125 w1156] -> w1113
                            tunnel: [w1126 w1155] -> w1112
                            tunnel: w1111 -> [w1128 w1154]
                            tunnel: w1110 -> [w1127 w1153]
                            tunnel: w1109 -> [w1121 w1151]
                            tunnel: w1108 -> [_ w1150]
                            tunnel: w1107 -> [w1122 w1149]
                            tunnel: [w1130 w1148] -> w1106
                            tunnel: w1105 -> [w1119 w1146]
                            tunnel: w1104 -> [w1120 w1145]
                            tunnel: w1103 -> [_ w1144]
                            tunnel: [w1129 w1143] -> w1102
                            frame 0 {
                              n323 = call "Corrected current calculator (SubVI).vi"("Necessary current"=w1122, "I_set old"=w1122, "Actual current"=w1121) -> ("I_set new"=w1130:dbl)  [unwired: 8 in]
                              n324 = call "Corrected current calculator (SubVI).vi"("Necessary current"=w1124, "I_set old"=w1124, "Actual current"=w1123) -> ("I_set new"=w1131:dbl)  [unwired: 8 in]
                              n325 = call "Corrected current calculator (SubVI).vi"("Necessary current"=w1120, "I_set old"=w1120, "Actual current"=w1119) -> ("I_set new"=w1129:dbl)  [unwired: 8 in]
                              n326 = Number To Fractional String(number=w1131) -> (F-format string=w1138:string)  [unwired: 3 in]
                              n327 = Number To Fractional String(number=w1130) -> (F-format string=w1136:string)  [unwired: 3 in]
                              n328 = Number To Fractional String(number=w1129) -> (F-format string=w1135:string)  [unwired: 3 in]
                              n329 = call "Set I2 (SubVI).vi"("Current Y"=w1136) -> ("String"=w1133:string)  [unwired: 10 in]
                              n330 = call "Set I1 (SubVI).vi"("Current X"=w1138) -> ("String instruction"=w1132:string)  [unwired: 10 in]
                              n331 = call "Set I3 (SubVI).vi"("Current Z"=w1135) -> ("String"=w1134:string)  [unwired: 10 in]
                              n332 = Concatenate Strings(w1132, w1133, w1134) -> (w1137:string)
                              n333 = VISA Write(VISA resource name=w1128, write buffer=w1137, error in (no error)=w1127) -> (VISA resource name out=w1125:refnum<visa-resource-name>, error out=w1126:errorcluster)  [unwired: 1 out]
                            }
                            frame Default {
                              # "Correct currents: calculate the new necessary current value; send the new current value to the power supply; place this newt I set on the while loop shift register."
                              n334 = call "Corrected current calculator (SubVI).vi"("Necessary current"=w1149, "I_set old"=w1150, "Actual current"=w1151) -> ("I_set new"=w1148:dbl)  [unwired: 8 in]
                              n335 = call "Corrected current calculator (SubVI).vi"("Necessary current"=w1159, "I_set old"=w1160, "Actual current"=w1161) -> ("I_set new"=w1158:dbl)  [unwired: 8 in]
                              n336 = call "Corrected current calculator (SubVI).vi"("Necessary current"=w1145, "I_set old"=w1144, "Actual current"=w1146) -> ("I_set new"=w1143:dbl)  [unwired: 8 in]
                              n337 = Number To Fractional String(number=w1158) -> (F-format string=w1157:string)  [unwired: 3 in]
                              n338 = Number To Fractional String(number=w1148) -> (F-format string=w1147:string)  [unwired: 3 in]
                              n339 = Number To Fractional String(number=w1143) -> (F-format string=w1142:string)  [unwired: 3 in]
                              n340 = call "Set I2 (SubVI).vi"("Current Y"=w1147) -> ("String"=w1140:string)  [unwired: 10 in]
                              n341 = call "Set I1 (SubVI).vi"("Current X"=w1157) -> ("String instruction"=w1139:string)  [unwired: 10 in]
                              n342 = call "Set I3 (SubVI).vi"("Current Z"=w1142) -> ("String"=w1141:string)  [unwired: 10 in]
                              n343 = Concatenate Strings(w1139, w1140, w1141) -> (w1152:string)
                              n344 = VISA Write(VISA resource name=w1154, write buffer=w1152, error in (no error)=w1153) -> (VISA resource name out=w1156:refnum<visa-resource-name>, error out=w1155:errorcluster)  [unwired: 1 out]
                            }
                          }
                          n345 = call "Z Coil Current to Magnetic field (SubVI).vi"("Current Z"=w1105) -> ("Magnetic field Z [µT]"=w1118:string)  [unwired: 10 in]
                          n346 = Wait (ms)(milliseconds to wait=u32 1000) -> ()  [unwired: 1 out]
                        }
                      }
                      n347 = Wait (ms)(milliseconds to wait=u32 500) -> ()  [unwired: 1 out]
                    }
                    n348 = feedback-in #16(w872) -> ()
                    n349 = feedback-in #17(w877) -> ()
                    n350 = feedback-in #18(w875) -> ()
                    n351 = call-poly <vilib>:"Write Delimited Spreadsheet.vi"("file path (dialog if empty)"=w884, "1D data"=w885, "append to file? (new file:F)"=TRUE, "delimiter (\\t)"="," ("delimiter (\\t)")) -> ()  [unwired: 10 in, 2 out]
                  }
                  n352 = feedback-in #13(w854) -> ()
                  n353 = feedback-in #14(w853) -> ()
                  n354 = feedback-in #15(w851) -> ()
                }
              }
            }
          }
        }
      }
    }
    n355 = VISA Close(VISA resource name=w8, error in (no error)=w7) -> (error out=w15:errorcluster)
    n356 = call <vilib>:"Simple Error Handler.vi"("error in (no error)"=w15) -> ()  [unwired: 1 in, 8 out]
  }
